vi "main 10th.vi"() -> ()   [LabVIEW 2015]
uses:
  Abort.vi
panel:
  out "OD Num 2":i32
  in  "Direct Summing Cluster":T1={"Direct Summing Path Na"="Nasum9", "Direct Summing Path Rb"="Rbsum9", "Enable Summing"=[FALSE, FALSE]}
  out "number of function calls":i32=187
  out "External Trigger":bool
  out "x-y":u32
  in  "Live Image Display 2":refnum<k7>(container)
  in  "Live Image Display":refnum<k7>(container)
  in  "Initial guess values 2":dbl[](array[numeric])
  in  "Fitting Results Save Path 2":string[](array[string])
  out "Current File Num":u16
  out "Two Cameras ?":bool
  out "3":u32=2150809629
  out "2":u32=2150809629
  out "5":u32=2150809629
  out "4":u32=2150809629
  out "From OD fit?":bool
  in  "Fitting Results Save Path":string[](array[string])
  in  "Initial guess values":dbl[](array[numeric])
  out "Latest image data":dbl[][](array[numeric])
  in  "Fitting Type":u16(ring)
  in  "Force Guess?":bool
  in  "Tab Control":enum32{"Page 1", "Page 2"}(tab)
  in  "Na Fitting ROI":T2
  in  "Rb Fitting ROI":T2
  in  "Get Image":bool
  in  "Open Na/Rb":u16(ring)=1 items=["Na", "Rb"]
  in  "Na/Rb (0/1)":u8(ring) items=["Na", "Rb"]
  in  "Abort":bool
  in  "FFT Auto?":bool[](array[boolean])=[FALSE, FALSE] caption="Auto?"
  in  "Ring":u16(ring)=3 items=["Atom", "Light", "Dark", "OD"]
  in  "Select Cam Fit":bool[](array[boolean])=[FALSE, FALSE]
  in  "Binning Average?":bool caption="Average?"
  in  "FFT Process":bool caption="Process"
  in  "Threshold":dbl
  out "Label":string[](array[string])=["Peak", "Xc", "Yc", "SigX", "SigY", "Offset"]
  in  "Pics to show in IJ":bool[][](array[boolean])=[[FALSE, FALSE], [FALSE, FALSE], [FALSE, FALSE], [TRUE, TRUE]]
  out "Trigger":bool
  in  "Save Fit":bool
  out "best fit parameters 2":dbl[][](array[numeric])
  in  "Binning Enabled":bool=TRUE
  in  "Binning":u8[](array[numeric])=[2, 2]
  out "ROI Width":u16[](array[numeric])
  out "ROI Height":u16[](array[numeric])
  out "best fit parameters":dbl[][](array[numeric])
  in  "Reset Cam Buffer":bool
  out "OD image":dbl[][](graph)
  out "Vertical Fitting":cluster{i32[], dbl[]}[](graph)
  in  "OD fit":bool caption="Open"
  in  "OD Num":i32
  out "Fitting...":bool
  in  "Exit":bool
  out "Horizontal Fitting":cluster{i32[], dbl[]}[](graph)=[{[0, 1, 2, 3, 4, 5, 6, 7, 8, 9, 10, 11, 12, 13, 14, 15, 16, 17, 18, 19, 20, 21, 22, 23, 24, 25, 26, 27, 28, 29, 30, 31, 32, 33, 34, 35, 36, 37, 38, 39, 40, 41, 42, 43, 44, 45, 46, 47, 48, 49, 50, 51, 52, 53, 54, 55, 56, 57, 58, 59, 60, 61, 62, 63, 64, 65, 66, 67, 68, 69, 70, 71, 72, 73, 74, 75, 76, 77, 78, 79, 80, 81, 82, 83, 84, 85, 86, 87, 88, 89, 90, 91, 92, 93, 94, 95, 96, 97, 98, 99, 100, 101, 102, 103, 104, 105, 106, 107, 108, 109, 110, 111, 112, 113, 114, 115, 116, 117, 118, 119, 120, 121, 122, 123, 124, 125, 126, 127, 128, 129, 130, 131, 132, 133, 134, 135, 136, 137, 138, 139, 140, 141, 142, 143, 144, 145, 146, 147, 148, 149, 150, 151, 152, 153, 154, 155, 156, 157, 158, 159, 160, 161, 162, 163, 164, 165, 166, 167, 168, 169, 170, 171, 172, 173, 174, 175, 176, 177, 178, 179, 180, 181, 182, 183, 184, 185, 186, 187, 188, 189, 190, 191, 192, 193, 194, 195, 196, 197, 198, 199], [271.0, 251.0, 239.0, 241.0, 236.0, 262.0, 271.0, 264.0, 266.0, 276.0, 292.0, 228.0, 254.0, 281.0, 219.0, 235.0, 280.0, 281.0, 291.0, 273.0, 299.0, 232.0, 255.0, 240.0, 222.0, 240.0, 240.0, 279.0, 296.0, 297.0, 339.0, 331.0, 313.0, 319.0, 271.0, 292.0, 320.0, 329.0, 342.0, 366.0, 378.0, 346.0, 370.0, 337.0, 334.0, 380.0, 391.0, 444.0, 455.0, 496.0, 509.0, 523.0, 587.0, 603.0, 674.0, 719.0, 851.0, 957.0, 1087.0, 1198.0, 1344.0, 1496.0, 1728.0, 1883.0, 2195.0, 2355.0, 2618.0, 2793.0, 3092.0, 3461.0, 3553.0, 3556.0, 3917.0, 4123.0, 4392.0, 4166.0, 4433.0, 4167.0, 4185.0, 3907.0, 3845.0, 3513.0, 3349.0, 3193.0, 2986.0, 2742.0, 2439.0, 2364.0, 2228.0, 2124.0, 2115.0, 1979.0, 1826.0, 1691.0, 1515.0, 1349.0, 1218.0, 1097.0, 1000.0, 932.0, 787.0, 729.0, 689.0, 578.0, 552.0, 477.0, 513.0, 476.0, 454.0, 434.0, 426.0, 416.0, 377.0, 352.0, 301.0, 326.0, 343.0, 299.0, 311.0, 312.0, 333.0, 330.0, 327.0, 244.0, 229.0, 253.0, 246.0, 250.0, 212.0, 284.0, 270.0, 266.0, 272.0, 267.0, 277.0, 267.0, 251.0, 272.0, 266.0, 265.0, 217.0, 267.0, 275.0, 261.0, 260.0, 253.0, 240.0, 211.0, 261.0, 288.0, 216.0, 259.0, 250.0, 263.0, 252.0, 231.0, 253.0, 269.0, 246.0, 219.0, 238.0, 279.0, 310.0, 259.0, 238.0, 270.0, 237.0, 224.0, 265.0, 263.0, 237.0, 243.0, 236.0, 287.0, 272.0, 238.0, 270.0, 249.0, 228.0, 276.0, 254.0, 251.0, 258.0, 284.0, 232.0, 275.0, 264.0, 230.0, 206.0, 247.0, 249.0, 299.0, 232.0, 226.0, 274.0, 258.0, 228.0, 237.0, 226.0, 272.0]}, {[0, 1, 2, 3, 4, 5, 6, 7, 8, 9, 10, 11, 12, 13, 14, 15, 16, 17, 18, 19, 20, 21, 22, 23, 24, 25, 26, 27, 28, 29, 30, 31, 32, 33, 34, 35, 36, 37, 38, 39, 40, 41, 42, 43, 44, 45, 46, 47, 48, 49, 50, 51, 52, 53, 54, 55, 56, 57, 58, 59, 60, 61, 62, 63, 64, 65, 66, 67, 68, 69, 70, 71, 72, 73, 74, 75, 76, 77, 78, 79, 80, 81, 82, 83, 84, 85, 86, 87, 88, 89, 90, 91, 92, 93, 94, 95, 96, 97, 98, 99, 100, 101, 102, 103, 104, 105, 106, 107, 108, 109, 110, 111, 112, 113, 114, 115, 116, 117, 118, 119, 120, 121, 122, 123, 124, 125, 126, 127, 128, 129, 130, 131, 132, 133, 134, 135, 136, 137, 138, 139, 140, 141, 142, 143, 144, 145, 146, 147, 148, 149, 150, 151, 152, 153, 154, 155, 156, 157, 158, 159, 160, 161, 162, 163, 164, 165, 166, 167, 168, 169, 170, 171, 172, 173, 174, 175, 176, 177, 178, 179, 180, 181, 182, 183, 184, 185, 186, 187, 188, 189, 190, 191, 192, 193, 194, 195, 196, 197, 198, 199], [258.6806156316728, 258.6716342989377, 258.6626530747521, 258.6536720452062, 258.644691361713, 258.6357112882564, 258.6267322810702, 258.61775512175285, 258.608781137568, 258.59981256259033, 258.5908531241233, 258.58190898580693, 258.57299024978414, 258.56411332615136, 258.5553046339484, 258.54660632509234, 258.53808504915014, 258.5298452400012, 258.5220490536178, 258.5149459806351, 258.5089163736844, 258.50453475825293, 258.5026609419198, 258.50456971619576, 258.5121334787082, 258.52807650614886, 258.556324973247, 258.6024831881351, 258.67447387274734, 258.78338851820223, 258.94460259167346, 259.17921915836735, 259.51591254856515, 259.993249982826, 260.6625721744371, 261.5915121253092, 262.86822258072306, 264.606364643175, 266.95088051361154, 270.08453000321674, 274.2351115263941, 279.6832126987842, 286.77024355158215, 295.9063984703781, 307.5780750260748, 322.3541549900494, 340.8904336545859, 363.9313792544649, 392.3083281288412, 426.93318811176084, 468.7867478105236, 518.9007873197883, 578.3333683044344, 648.1369555436747, 729.3193888427367, 822.7981764748481, 929.3491024699478, 1049.550703700878, 1183.72674293613, 1331.889336934238, 1493.6858449827125, 1668.352932109982, 1854.6813445196683, 2050.994832619432, 2255.1463024696804, 2464.533660376819, 2676.1369496341113, 2886.5772978639948, 3092.1969553318745, 3289.15838608278, 3473.5590667034103, 3641.557451626854, 3789.5045781946988, 3914.0750983875137, 4012.3912077845603, 4082.133040191528, 4121.629620994105, 4129.925401766357, 4106.818677312171, 4052.869728621802, 3969.378232753251, 3858.331211349985, 3722.32442841007, 3564.4615781318566, 3388.236726522453, 3197.4062138342942, 2995.8565487684205, 2787.4747242211, 2576.026886168148, 2365.0504495856335, 2157.7636585036757, 1956.9953263662687, 1765.1361682792287, 1584.1118454713421, 1415.3766700512429, 1259.925933154814, 1118.3240687125547, 990.7453722391384, 877.0237608957168, 776.70806955959, 689.1195940765085, 613.4089728479037, 548.609991424882, 493.6884511769152, 447.5848152437265, 409.24989248464567, 377.67331147174724, 351.90494998495853, 331.0698089332847, 314.3770499408072, 301.12405712687945, 290.6964455185657, 282.56493430017093, 276.2799477549777, 271.46471553103595, 267.80753099497196, 265.05370427973, 262.9976251657801, 261.47523759206035, 260.3571273330433, 259.54233995504075, 258.9529785017419, 258.5295789767464, 258.2272251324483, 258.01234029108025, 257.8600805980793, 257.75224890635894, 257.6756492398139, 257.6208065847789, 257.5809840355968, 257.55143783992105, 257.5288597354012, 257.5109645077476, 257.49618853007837, 257.4834719474245, 257.47210306669035, 257.4616084138856, 257.45167589964194, 257.44210169672607, 257.4327538988841, 257.42354791849357, 257.4144300024347, 257.4053662996607, 257.3963356836851, 257.3873250872788, 257.37832650004066, 257.3693350550716, 257.3603478215476, 257.3513630501138, 257.34237970580045, 257.3333971816626, 257.32441512488083, 257.3154333321509, 257.306451687344, 257.29747012470295, 257.2884886073164, 257.2795071146445, 257.2705256353558, 257.26154416325335, 257.25256269497714, 257.24358122872104, 257.23459976352257, 257.2256182988732, 257.21663683450635, 257.2076553702838, 257.19867390613433, 257.1896924420215, 257.18071097792694, 257.17172951384134, 257.16274804976024, 257.15376658568124, 257.1447851216032, 257.13580365752574, 257.12682219344845, 257.11784072937127, 257.10885926529426, 257.09987780121713, 257.09089633714007, 257.081914873063, 257.07293340898593, 257.06395194490887, 257.0549704808318, 257.0459890167548, 257.0370075526777, 257.02802608860065, 257.0190446245236, 257.0100631604465, 257.00108169636945, 256.9921002322924, 256.9831187682154, 256.9741373041383, 256.96515584006124, 256.9561743759842, 256.9471929119071, 256.93821144783004, 256.92922998375303, 256.92024851967597, 256.9112670555989, 256.90228559152183, 256.89330412744476]}]
  in  "Fit":bool
  in  "Open File":bool
  in  "Auto Fit":bool
  in  "Stop":bool
  in  "Aquire":bool
  in  "Fitting Config":bool
  in  "Camera Config":bool
  in  "Initialize":bool
  # "Cam1"
  # "Cam2"
  # "Atom"
  # "Light"
  # "Dark"
  # "OD"
  # "FFT and Low Pass"
  # "Na"
  # "Rb"
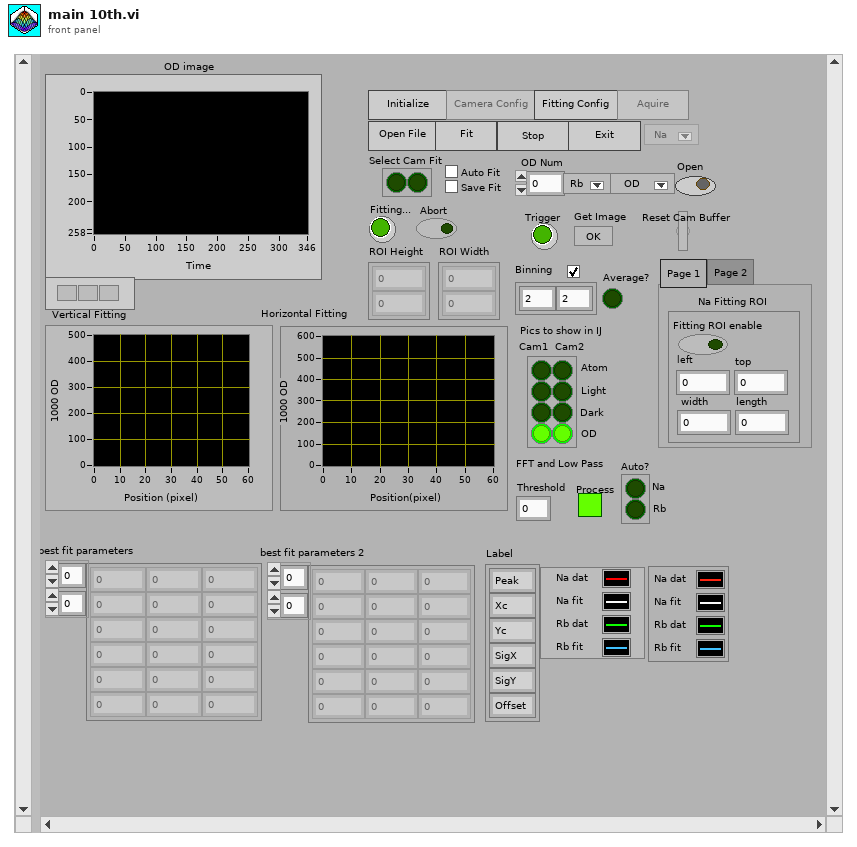
[diagram p1: front panel]
types:
  T1 = cluster{"Direct Summing Path Na":string, "Direct Summing Path Rb":string, "Enable Summing":bool[]}
  T2 = cluster{"Fitting ROI enable":bool, "top":i32, "length":i32, "left":i32, " width":i32}
  T3 = enum8{"Enabled", "Disabled", "Disabled and Grayed Out"}
  T4 = enum16{"Left Button", "Center Button", "Right Button", "Window Close"}
  T5 = typedef "Image Type" = u32
  T6 = typedef "IMAQ Image.ctl" = refnum<image>
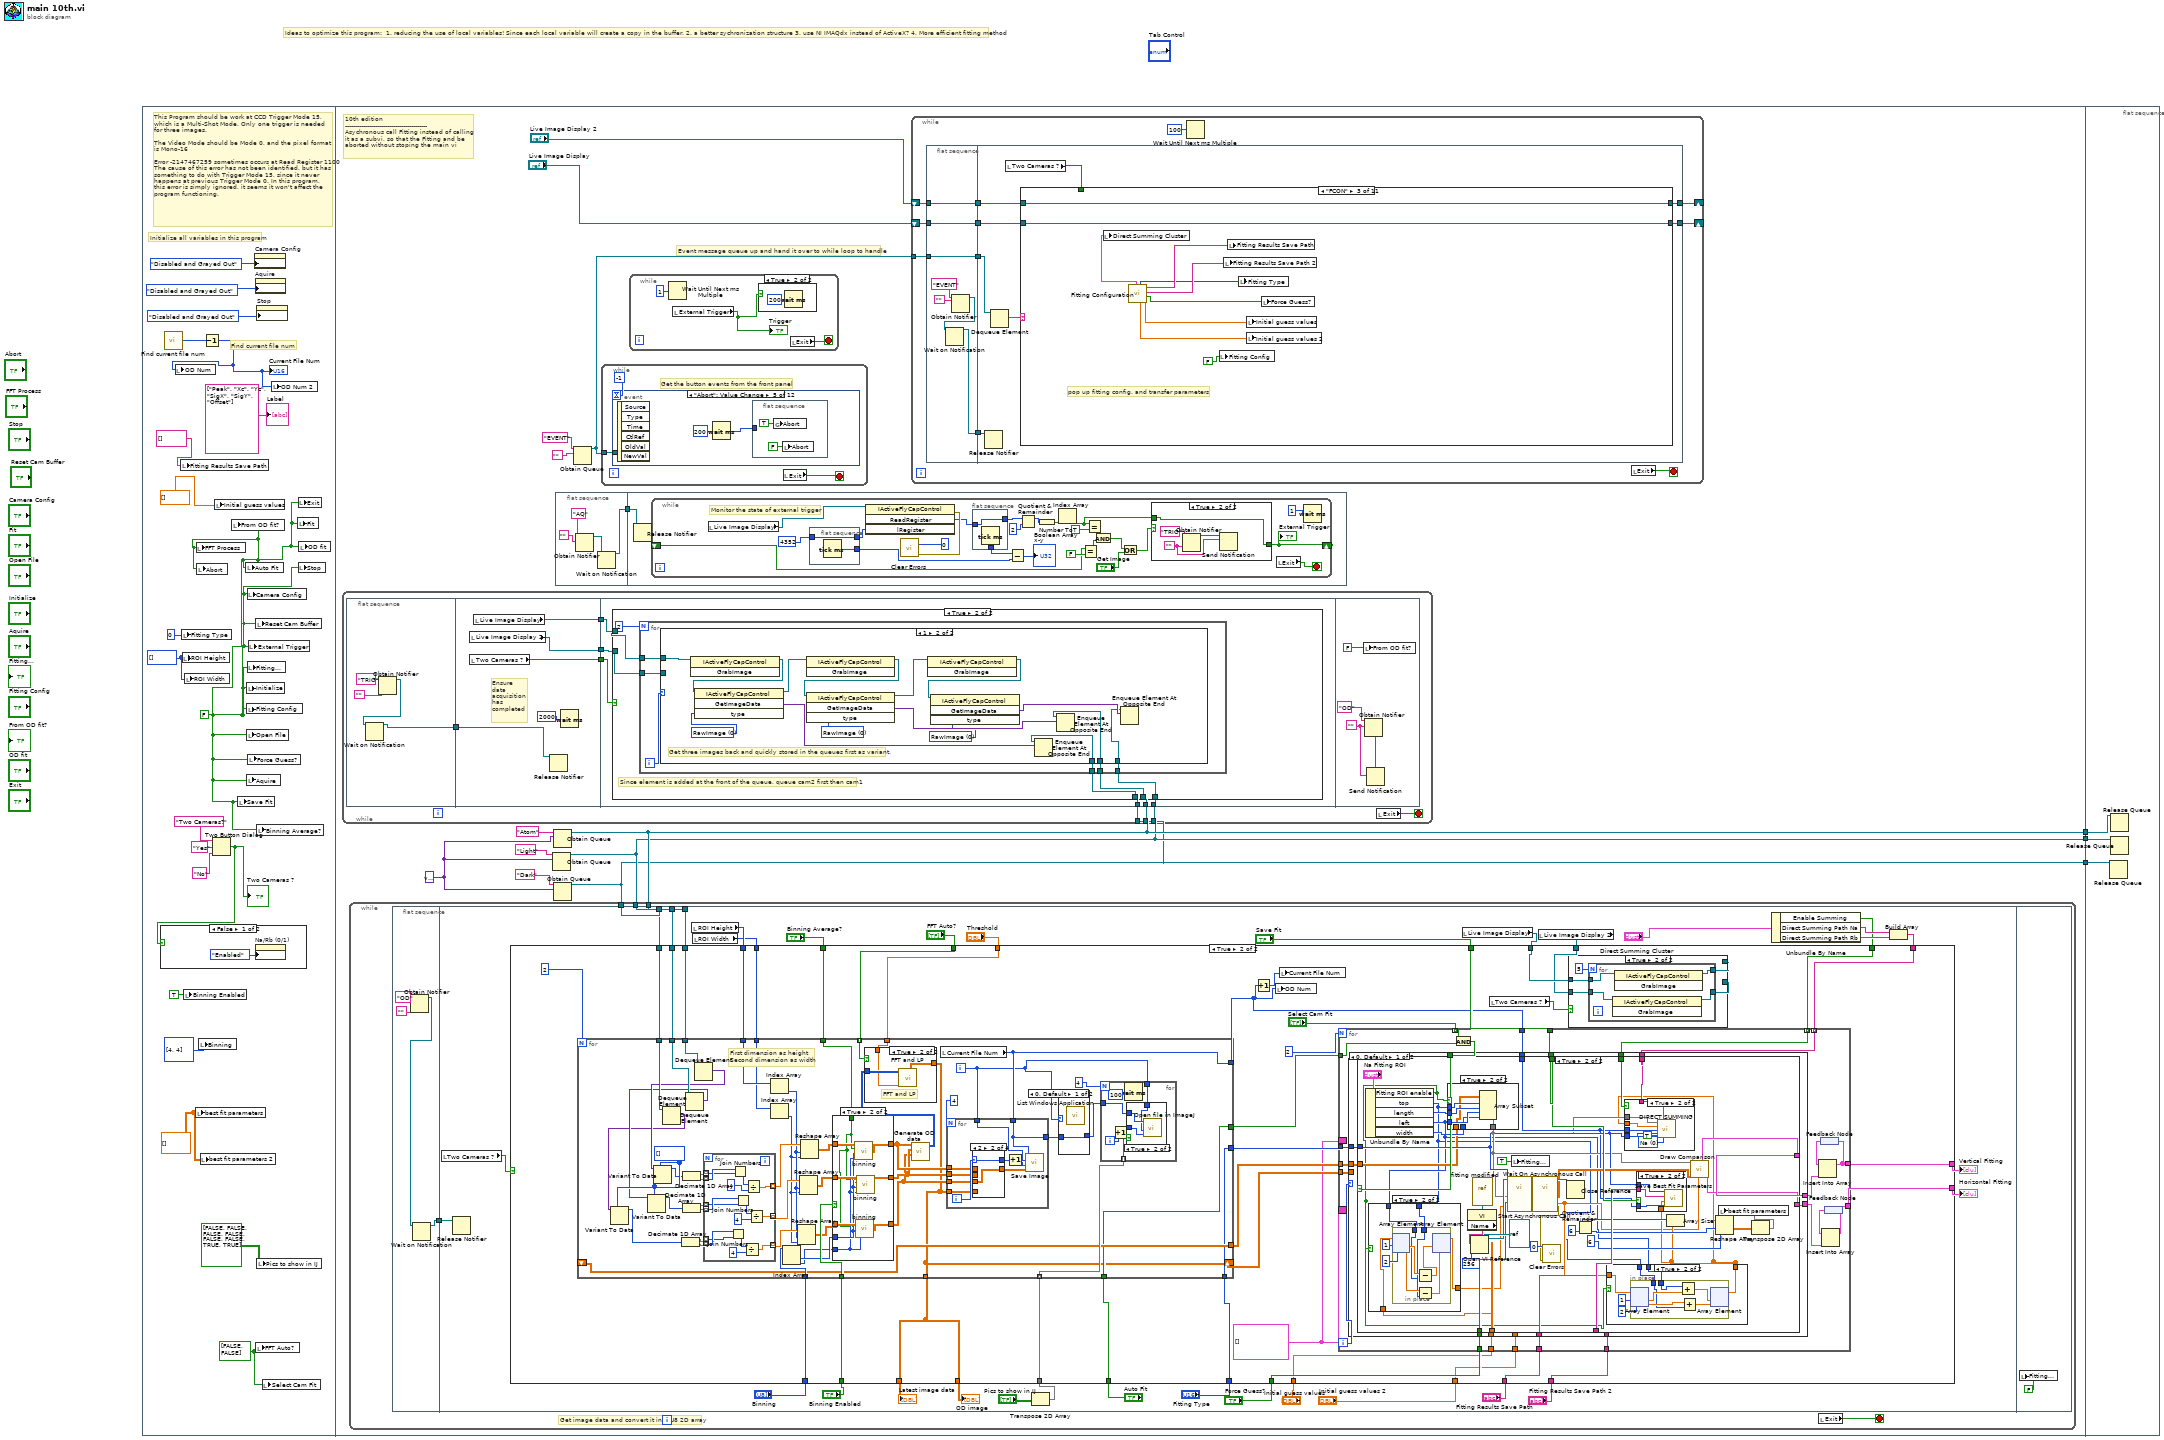
[diagram p0: block diagram]
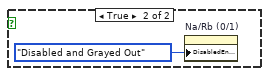
[diagram p2: hidden frame]
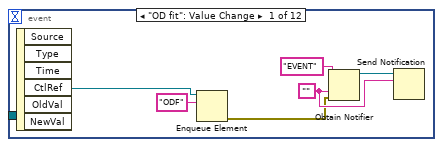
[diagram p4: hidden frame]
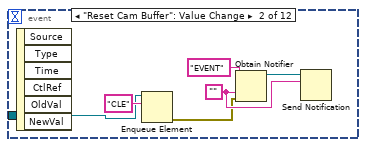
[diagram p5: hidden frame]
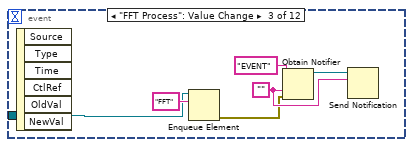
[diagram p6: hidden frame]
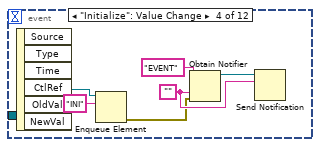
[diagram p7: hidden frame]
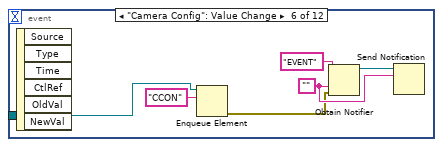
[diagram p8: hidden frame]
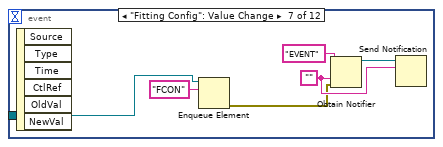
[diagram p9: hidden frame]
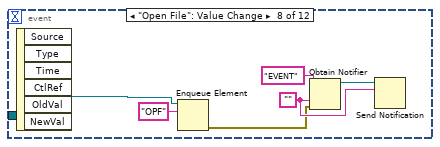
[diagram p10: hidden frame]
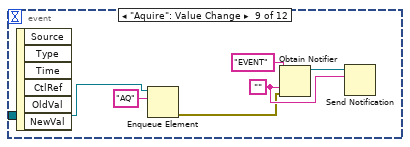
[diagram p11: hidden frame]
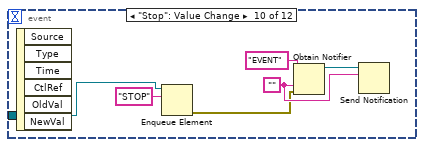
[diagram p12: hidden frame]
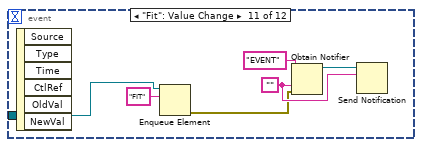
[diagram p13: hidden frame]
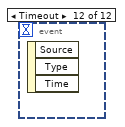
[diagram p14: hidden frame]
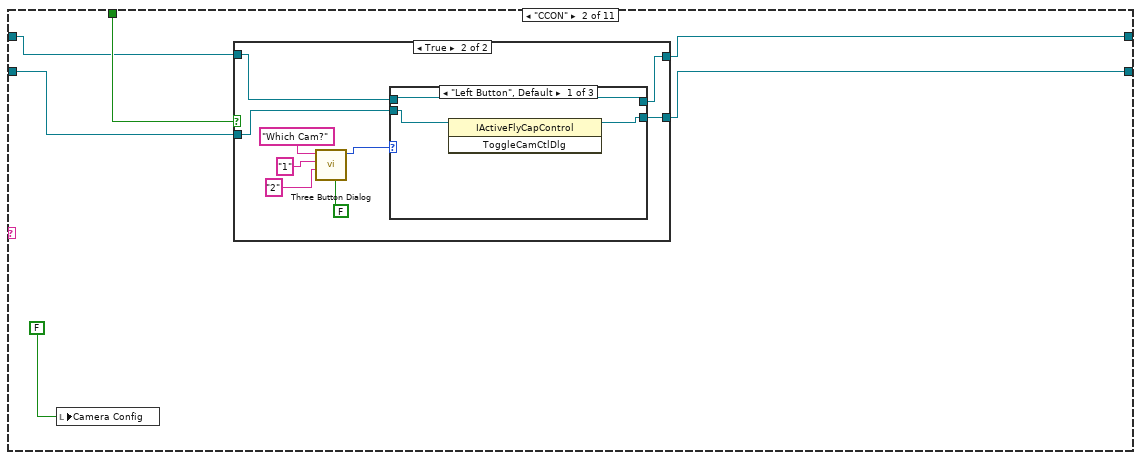
[diagram p16: hidden frame]
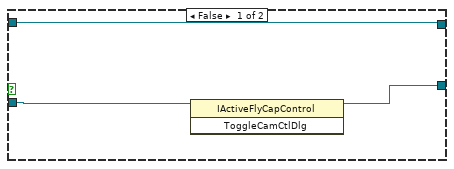
[diagram p17: hidden frame]
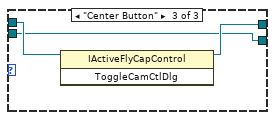
[diagram p19: hidden frame]
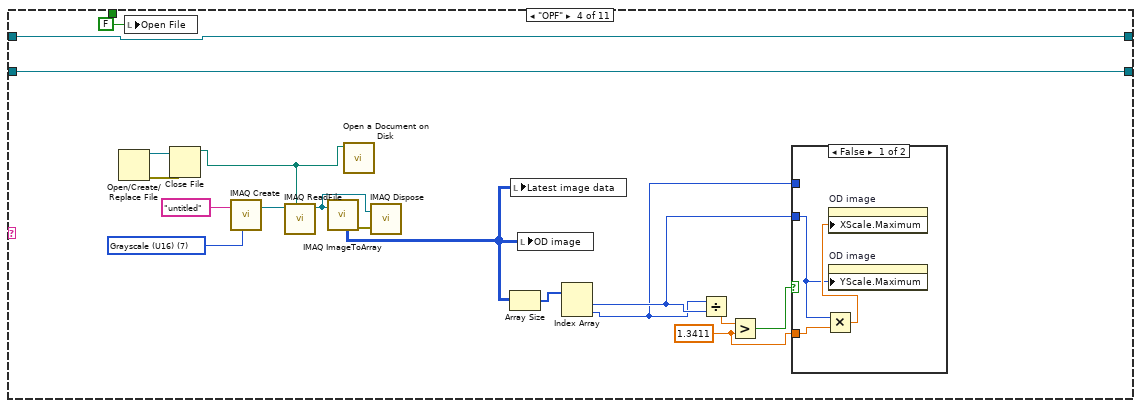
[diagram p20: hidden frame]
diagram:
  # "Ideas to optimize this program:  1. reducing the use of local variables! Since each local variable will create a copy in the buffer. 2. a better sychronization structure 3. use NI IMAQdx instead of ActiveX? 4. More efficient fitting method"
  n1 = flat-sequence {
    tunnel: [w34] -> w3
    tunnel: [w33] -> w2
    tunnel: [w32] -> w1
    tunnel: w3 -> [w1227]
    tunnel: w2 -> [w1226]
    tunnel: w1 -> [w1225]
    frame #0 {
      w5 = bool[] [FALSE, FALSE] ("FFT Auto?")
      w10 = dbl[][] [] ("best fit parameters")
      w14 = u16[] [] ("ROI Height")
      w8 = FALSE ("Aquire")
      # "This Program should be work at CCD Trigger Mode 15,\nwhich is a Multi-Shot Mode. Only one trigger is needed\nfor three images. \n\nThe Video Mode should be Mode 0, and the pixel format\nis Mono-16\n\nError -2147467259 sometimes occurs at Read Register 1100\nThe cause of this error has not been identified, but it has\nsomething to do with Trigger Mode 15, since it never \nhappens at previous Trigger Mode 0. In this program,\nthis error is simply ignored, it seems it won't affect the \nprogram functioning."
      # "Find current file num"
      # "Initialize all variables in this program"
      n2 = call "Find current file num.vi"() -> ("Current File Num"=w9:u16)  [unwired: 2 in]
      n3 = local write "Fitting Results Save Path"(string[] [] ("Fitting Results Save Path")) -> ()
      n4 = local write "Fitting Type"(0 ("OD num")) -> ()
      n5 = local write "ROI Height"(w14) -> ()
      n6 = local write "Binning Enabled"(TRUE ("Binning Enabled")) -> ()
      n7 = local write "ROI Width"(w14) -> ()
      n8 = local write "best fit parameters"(w10) -> ()
      n9 = local write "FFT Process"(w8) -> ()
      n10 = local write "Abort"(w8) -> ()
      n11 = local write "Binning"(u8[] [4, 4] ("Binning")) -> ()
      n12 = local write "best fit parameters 2"(w10) -> ()
      n13 = Decrement(x=w9) -> (x-1=w4:u16)
      "Current File Num" <- w4
      n14 = local write "OD Num"(w4) -> ()
      n15 = Two Button Dialog(message="Two Cameras?" ("消息"), 1:"No" ("F按钮名称（“取消”）"), 2:"Yes" ("T按钮名称（“确定”）")) -> (T button?=w7:bool)
      "Two Cameras ?" <- w7
      n16 = case shown="False" w7 {
        frame False {
          n17 = property on="Na/Rb (0/1)" class="Ring (strict)"("DisabledEnum"=T3."Enabled" ("Disabled")) -> ()  [unwired: 2 in, 2 out]
        }
        frame True {
          n18 = property on="Na/Rb (0/1)" class="Ring (strict)"("DisabledEnum"=T3."Disabled and Grayed Out" ("Disabled")) -> ()  [unwired: 2 in, 2 out]
        }
      }
      n19 = local write "Initial guess values"(dbl[] [] ("Best fit parameters")) -> ()
      n20 = local write "From OD fit?"(w8) -> ()
      n21 = local write "Save Fit"(w8) -> ()
      n22 = local write "Auto Fit"(w8) -> ()
      n23 = local write "Initialize"(w8) -> ()
      n24 = local write "Fitting Config"(w8) -> ()
      n25 = local write "Open File"(w8) -> ()
      n26 = local write "Aquire"(w8) -> ()
      n27 = local write "Camera Config"(w8) -> ()
      n28 = local write "Fitting..."(w8) -> ()
      n29 = local write "Force Guess?"(w8) -> ()
      n30 = local write "External Trigger"(w8) -> ()
      n31 = property on="Camera Config" class="Bool (strict)"("DisabledEnum"=T3."Disabled and Grayed Out" ("禁用")) -> ()  [unwired: 2 in, 2 out]
      n32 = property on="Aquire" class="Bool (strict)"("DisabledEnum"=T3."Disabled and Grayed Out" ("禁用")) -> ()  [unwired: 2 in, 2 out]
      n33 = local write "Reset Cam Buffer"(w8) -> ()
      n34 = local write "FFT Auto?"(w5) -> ()
      n35 = local write "Binning Average?"(w8) -> ()
      n36 = property on="Stop" class="Bool (strict)"("DisabledEnum"=T3."Disabled and Grayed Out" ("禁用")) -> ()  [unwired: 2 in, 2 out]
      n37 = local write "Pics to show in IJ"(bool[][] [[FALSE, FALSE], [FALSE, FALSE], [FALSE, FALSE], [TRUE, TRUE]] ("Pics to show in IJ")) -> ()
      n38 = local write "Select Cam Fit"(w5) -> ()
      n39 = local write "OD Num 2"(w4) -> ()
      n40 = local write "Fit"(w8) -> ()
      n41 = local write "Exit"(w8) -> ()
      n42 = local write "Stop"(w8) -> ()
      n43 = local write "OD fit"(w8) -> ()
      "Label" <- string[] ["Peak", "Xc", "Yc", "SigX", "SigY", "Offset"] ("Label")
    }
    frame #1 {
      w28 = variant
      # "10th edition\n-----------------------------------------\nAsychronous call Fitting instead of calling\nit as a subvi, so that the Fitting and be \naborted without stoping the main vi"
      # "Event message queue up and hand it over to while loop to handle"
      n44 = Obtain Queue(name (unnamed)="Light" ("名称（未命名）"), element data type=w28) -> (queue out=w33:refnum<queue>)  [unwired: 3 in, 2 out]
      n45 = Obtain Queue(name (unnamed)="Atom" ("名称（未命名）"), element data type=w28) -> (queue out=w34:refnum<queue>)  [unwired: 3 in, 2 out]
      n46 = Obtain Queue(name (unnamed)="Dark" ("名称（未命名）"), element data type=w28) -> (queue out=w32:refnum<queue>)  [unwired: 3 in, 2 out]
      n47 = while {
        tunnel: w34 -> [w1135]
        tunnel: w33 -> [w1134]
        tunnel: w32 -> [w1133]
        stop <- w1129 stop-if-true
        n48 = flat-sequence {
          tunnel: [w1137] -> w1136
          tunnel: w1136 -> [w1145]
          tunnel: [w1144] -> w1132
          tunnel: [w1143] -> w1131
          tunnel: [w1142] -> w1130
          tunnel: w1135 -> [w1151]
          tunnel: w1134 -> [w1150]
          tunnel: w1133 -> [w1149]
          tunnel: w1132 -> [w1148]
          tunnel: w1131 -> [w1147]
          tunnel: w1130 -> [w1146]
          frame #0 {
            n49 = Obtain Notifier(name (unnamed)="TRIG" ("名称（未命名）"), notification data type="") -> (notifier out=w1138:refnum<notifier>)  [unwired: 2 in, 2 out]
            n50 = Wait on Notification(notifier=w1138) -> (notifier out=w1137:refnum<notifier>)  [unwired: 3 in, 3 out]
          }
          frame #1 {
            # "Ensure\ndata\nacquisition\nhas \ncompleted"
            n51 = local read "Live Image Display 2"() -> (w1143:refnum<k7>)
            n52 = local read "Two Cameras ?"() -> (w1142:bool)
            n53 = local read "Live Image Display"() -> (w1144:refnum<k7>)
            n54 = Release Notifier(notifier=w1145) -> ()  [unwired: 2 in, 3 out]
            n55 = Wait (ms)(milliseconds to wait=u32 2000) -> ()  [unwired: 1 out]
          }
          frame #2 {
            n56 = case shown="True" w1146 {
              tunnel: w1151 -> [w1169 w1184]
              tunnel: w1150 -> [w1160 w1183]
              tunnel: w1149 -> [w1157 w1182]
              tunnel: w1148 -> [w1153 w1180]
              tunnel: w1147 -> [_ w1179]
              frame False {
                w1155 = 0 items=["RawImage", "ColorProcessedImage"] ("type")
                w1156 = 0 items=["RawImage", "ColorProcessedImage"] ("type")
                w1170 = 0 items=["RawImage", "ColorProcessedImage"] ("type")
                # "Get three images back and quickly stored in the queues first as variant."
                n57 = invoke class="IActiveFlyCapControl" method="GrabImage"(reference=w1153) -> (reference out=w1152:refnum<k7>)  [unwired: 2 in, 2 out]
                n58 = flat-sequence {
                  tunnel: w1152 -> [w1173]
                  tunnel: [w1173] -> w1167
                  frame #0 {
                    n59 = Tick Count (ms)() -> (millisecond timer value=→"2":u32)
                  }
                }
                n60 = invoke class="IActiveFlyCapControl" method="GetImageData"(reference=w1167, "type"=w1170) -> (reference out=w1164:refnum<k7>, "GetImageData"=w1166:variant)  [unwired: 2 in, 2 out]
                n61 = invoke class="IActiveFlyCapControl" method="GrabImage"(reference=w1164) -> (reference out=w1163:refnum<k7>)  [unwired: 2 in, 2 out]
                n62 = flat-sequence {
                  tunnel: [w1171] -> w1165
                  tunnel: w1166 -> [w1171]
                  frame #0 {
                    n63 = Tick Count (ms)() -> (millisecond timer value=→"3":u32)
                  }
                }
                n64 = invoke class="IActiveFlyCapControl" method="GetImageData"(reference=w1163, "type"=w1156) -> (reference out=w1162:refnum<k7>, "GetImageData"=w1161:variant)  [unwired: 2 in, 2 out]
                n65 = flat-sequence {
                  tunnel: w1165 -> [w1178]
                  tunnel: [w1178] -> w1168
                  frame #0 {
                    n66 = Tick Count (ms)() -> (millisecond timer value=→"4":u32)
                  }
                }
                n67 = invoke class="IActiveFlyCapControl" method="GrabImage"(reference=w1162) -> (reference out=w1159:refnum<k7>)  [unwired: 2 in, 2 out]
                n68 = Enqueue Element At Opposite End(queue=w1169, element=w1168) -> ()  [unwired: 2 in, 3 out]
                n69 = Enqueue Element At Opposite End(queue=w1160, element=w1161) -> ()  [unwired: 2 in, 3 out]
                n70 = invoke class="IActiveFlyCapControl" method="GetImageData"(reference=w1159, "type"=w1155) -> ("GetImageData"=w1158:variant)  [unwired: 2 in, 3 out]
                n71 = flat-sequence {
                  tunnel: w1157 -> [w1175]
                  tunnel: [w1175] -> w1154
                  frame #0 {
                    n72 = Tick Count (ms)() -> (millisecond timer value=→"5":u32)
                  }
                }
                n73 = Enqueue Element At Opposite End(queue=w1154, element=w1158) -> ()  [unwired: 2 in, 3 out]
              }
              frame True {
                # "Since element is added at the front of the queue, queue cam2 first then cam1"
                n74 = for {
                  N: 2 -> [_]
                  tunnel: w1184 -> [w1190]
                  tunnel: w1183 -> [w1189]
                  tunnel: w1182 -> [w1188]
                  tunnel: w1180 -> [w1186]
                  tunnel: w1179 -> [w1185]
                  i -> [w1187]
                  n75 = case shown="1" w1187 {
                    tunnel: w1190 -> [w1194 w1210]
                    tunnel: w1189 -> [w1193 w1209]
                    tunnel: w1188 -> [w1192 w1208]
                    tunnel: w1186 -> [_ w1207]
                    tunnel: w1185 -> [w1191 _]
                    frame 0, Default {
                      w1197 = 0 items=["RawImage", "ColorProcessedImage"] ("type")
                      w1198 = 0 items=["RawImage", "ColorProcessedImage"] ("type")
                      w1205 = 0 items=["RawImage", "ColorProcessedImage"] ("type")
                      # "Get three images back and quickly stored in the queues first as variant."
                      n76 = invoke class="IActiveFlyCapControl" method="GrabImage"(reference=w1191) -> (reference out=w1196:refnum<k7>)  [unwired: 2 in, 2 out]
                      n77 = invoke class="IActiveFlyCapControl" method="GetImageData"(reference=w1196, "type"=w1205) -> (reference out=w1204:refnum<k7>, "GetImageData"=w1195:variant)  [unwired: 2 in, 2 out]
                      n78 = invoke class="IActiveFlyCapControl" method="GrabImage"(reference=w1204) -> (reference out=w1203:refnum<k7>)  [unwired: 2 in, 2 out]
                      n79 = invoke class="IActiveFlyCapControl" method="GetImageData"(reference=w1203, "type"=w1198) -> (reference out=w1202:refnum<k7>, "GetImageData"=w1201:variant)  [unwired: 2 in, 2 out]
                      n80 = invoke class="IActiveFlyCapControl" method="GrabImage"(reference=w1202) -> (reference out=w1200:refnum<k7>)  [unwired: 2 in, 2 out]
                      n81 = invoke class="IActiveFlyCapControl" method="GetImageData"(reference=w1200, "type"=w1197) -> ("GetImageData"=w1199:variant)  [unwired: 2 in, 3 out]
                      n82 = Enqueue Element At Opposite End(queue=w1194, element=w1195) -> ()  [unwired: 2 in, 3 out]
                      n83 = Enqueue Element At Opposite End(queue=w1193, element=w1201) -> ()  [unwired: 2 in, 3 out]
                      n84 = Enqueue Element At Opposite End(queue=w1192, element=w1199) -> ()  [unwired: 2 in, 3 out]
                    }
                    frame 1 {
                      w1213 = 0 items=["RawImage", "ColorProcessedImage"] ("type")
                      w1214 = 0 items=["RawImage", "ColorProcessedImage"] ("type")
                      w1220 = 0 items=["RawImage", "ColorProcessedImage"] ("type")
                      # "Get three images back and quickly stored in the queues first as variant."
                      n85 = invoke class="IActiveFlyCapControl" method="GrabImage"(reference=w1207) -> (reference out=w1212:refnum<k7>)  [unwired: 2 in, 2 out]
                      n86 = invoke class="IActiveFlyCapControl" method="GetImageData"(reference=w1212, "type"=w1220) -> (reference out=w1219:refnum<k7>, "GetImageData"=w1211:variant)  [unwired: 2 in, 2 out]
                      n87 = invoke class="IActiveFlyCapControl" method="GrabImage"(reference=w1219) -> (reference out=w1218:refnum<k7>)  [unwired: 2 in, 2 out]
                      n88 = invoke class="IActiveFlyCapControl" method="GetImageData"(reference=w1218, "type"=w1214) -> (reference out=w1217:refnum<k7>, "GetImageData"=w1216:variant)  [unwired: 2 in, 2 out]
                      n89 = invoke class="IActiveFlyCapControl" method="GrabImage"(reference=w1217) -> (reference out=w1206:refnum<k7>)  [unwired: 2 in, 2 out]
                      n90 = invoke class="IActiveFlyCapControl" method="GetImageData"(reference=w1206, "type"=w1213) -> ("GetImageData"=w1215:variant)  [unwired: 2 in, 3 out]
                      n91 = Enqueue Element At Opposite End(queue=w1210, element=w1211) -> ()  [unwired: 2 in, 3 out]
                      n92 = Enqueue Element At Opposite End(queue=w1209, element=w1216) -> ()  [unwired: 2 in, 3 out]
                      n93 = Enqueue Element At Opposite End(queue=w1208, element=w1215) -> ()  [unwired: 2 in, 3 out]
                    }
                  }
                }
              }
            }
          }
          frame #3 {
            w1222 = ""
            n94 = local write "From OD fit?"(FALSE ("From OD fit?")) -> ()
            n95 = Obtain Notifier(name (unnamed)="OD" ("名称（未命名）"), notification data type=w1222) -> (notifier out=w1224:refnum<notifier>)  [unwired: 2 in, 2 out]
            n96 = Send Notification(notification=w1222, notifier=w1224) -> ()  [unwired: 1 in, 2 out]
          }
        }
        n97 = local read "Exit"() -> (w1129:bool)
      }
      n98 = while {
        tunnel: w34 -> [w482]
        tunnel: w33 -> [w481]
        tunnel: w32 -> [w480]
        stop <- w479 stop-if-true
        # "Get image data and convert it into U8 2D array"
        n99 = flat-sequence {
          tunnel: [w484] -> w483
          tunnel: w483 -> [w517]
          tunnel: w482 -> [w520]
          tunnel: w481 -> [w519]
          tunnel: w480 -> [w518]
          frame #0 {
            n100 = Obtain Notifier(name (unnamed)="OD" ("名称（未命名）"), notification data type="") -> (notifier out=w485:refnum<notifier>)  [unwired: 2 in, 2 out]
            n101 = Wait on Notification(notifier=w485) -> (notifier out=w484:refnum<notifier>)  [unwired: 3 in, 3 out]
          }
          frame #1 {
            n102 = local read "Two Cameras ?"() -> (w516:bool)
            n103 = Release Notifier(notifier=w517) -> ()  [unwired: 2 in, 3 out]
            n104 = local read "ROI Height"() -> (w513:u16[])
            n105 = local read "ROI Width"() -> (w512:u16[])
            n106 = Transpose 2D Array(2D array="Pics to show in IJ") -> (transposed array=w499:bool[][])
            n107 = local read "Live Image Display"() -> (w495:refnum<k7>)
            n108 = local read "Live Image Display 2"() -> (w496:refnum<k7>)
            n109 = Unbundle By Name("Direct Summing Cluster") -> ("Enable Summing"=w489:bool[], "Direct Summing Path Na"=w491:string, "Direct Summing Path Rb"=w490:string)
            n110 = Build Array(w491, w490) -> (w488:string[])
            n111 = case shown="True" w516 {
              selector: w516 -> [w532 _]
              tunnel: w520 -> [w584 w744]
              tunnel: w519 -> [w583 w743]
              tunnel: w518 -> [w582 w742]
              tunnel: "Binning" -> [w551 w741]
              tunnel: "Binning Enabled" -> [w550 w740]
              tunnel: w513 -> [w549 w739]
              tunnel: w512 -> [w548 w738]
              tunnel: [w525 w737] -> w511
              tunnel: [w525 w737] -> w510
              tunnel: "Auto Fit" -> [w547 w736]
              tunnel: "Initial guess values" -> [w546 w725]
              tunnel: "Force Guess?" -> [w545 w726]
              tunnel: "Fitting Type" -> [w544 w735]
              tunnel: "Fitting Results Save Path" -> [w543 w722]
              tunnel: [w541 w718] -> w504
              tunnel: [w540 w717] -> w503
              tunnel: "Fitting Results Save Path 2" -> [_ w721]
              tunnel: "Initial guess values 2" -> [_ w720]
              tunnel: "Save Fit" -> [w539 w724]
              tunnel: w499 -> [w538 w733]
              tunnel: "Binning Average?" -> [w536 w732]
              tunnel: w496 -> [w534 w730]
              tunnel: w495 -> [w533 w731]
              tunnel: "Threshold" -> [w529 w714]
              tunnel: "FFT Auto?" -> [w531 w713]
              tunnel: w489 -> [w524 w709]
              tunnel: w488 -> [w522 w708]
              frame False {
                w567 = u8[] []
                # "FFT and LP"
                # "First dimension as height\nSecond dimension as width"
                # "use the current file num flow to control \nthe sequence, save first and then open files in IJ"
                n112 = Dequeue Element(queue=w582) -> (element=w565:variant)  [unwired: 2 in, 3 out]
                n113 = Variant To Data(type=w567, Variant=w565) -> (data=w562:u8[])  [unwired: 1 in, 1 out]
                n114 = Dequeue Element(queue=w583) -> (element=w566:variant)  [unwired: 2 in, 3 out]
                n115 = Variant To Data(type=w567, Variant=w566) -> (data=w563:u8[])  [unwired: 1 in, 1 out]
                n116 = Decimate 1D Array(w562) -> (w573:u8[], w572:u8[])
                n117 = Dequeue Element(queue=w584) -> (element=w568:variant)  [unwired: 2 in, 3 out]
                n118 = Variant To Data(type=w567, Variant=w568) -> (data=w564:u8[])  [unwired: 1 in, 1 out]
                n119 = Decimate 1D Array(w564) -> (w577:u8[], w576:u8[])
                n120 = Decimate 1D Array(w563) -> (w575:u8[], w574:u8[])
                n121 = for {
                  tunnel: [w631] -> w571 mode=indexing
                  tunnel: w577 -> [w621] mode=indexing
                  tunnel: w576 -> [w622] mode=indexing
                  tunnel: w575 -> [w623] mode=indexing
                  tunnel: w574 -> [w624] mode=indexing
                  tunnel: w573 -> [w625] mode=indexing
                  tunnel: w572 -> [w626] mode=indexing
                  tunnel: [w620] -> w570 mode=indexing
                  tunnel: [w619] -> w569 mode=indexing
                  n122 = Join Numbers(hi=w626, lo=w625) -> ((hi.lo)=w628:u16)
                  n123 = Join Numbers(hi=w622, lo=w621) -> ((hi.lo)=w633:u16)
                  n124 = Join Numbers(hi=w624, lo=w623) -> ((hi.lo)=w630:u16)
                  n125 = Divide(x=w628, y=u16 4) -> (x/y=w619:dbl)
                  n126 = Divide(x=w633, y=u16 4) -> (x/y=w631:dbl)
                  n127 = Divide(x=w630, y=u16 4) -> (x/y=w620:dbl)
                }
                n128 = Index Array(array=w548) -> (element=w560:u16)  [unwired: 1 in]
                n129 = Index Array(array=w549) -> (element=w561:u16)  [unwired: 1 in]
                n130 = Reshape Array(w569, w561, w560) -> (w554:dbl[][])
                n131 = Reshape Array(w570, w561, w560) -> (w556:dbl[][])
                n132 = Reshape Array(w571, w561, w560) -> (w558:dbl[][])
                n133 = Index Array(array=w551) -> (element #1=w553:u8, element #2=w552:u8)  [unwired: 2 in]
                n134 = case shown="True" w550 {
                  tunnel: [w609 w617] -> w559
                  tunnel: w558 -> [w609 w618]
                  tunnel: [w608 w615] -> w557
                  tunnel: w556 -> [w608 w616]
                  tunnel: [w607 w614] -> w555
                  tunnel: w554 -> [w607 w613]
                  tunnel: w553 -> [_ w612]
                  tunnel: w552 -> [_ w611]
                  tunnel: w536 -> [_ w610]
                  frame False {
                  }
                  frame True {
                    n135 = call "binning.vi"("y binning"=w611, "x binning"=w612, "Average?"=w610, "data in"=w618) -> ("data out"=w617:dbl[][])
                    n136 = call "binning.vi"("y binning"=w611, "x binning"=w612, "Average?"=w610, "data in"=w613) -> ("data out"=w614:dbl[][])
                    n137 = call "binning.vi"("y binning"=w611, "x binning"=w612, "Average?"=w610, "data in"=w616) -> ("data out"=w615:dbl[][])
                  }
                }
                n138 = Index Array(array=w531) -> (element=w530:bool)  [unwired: 1 in]
                n139 = call "Generate OD data.vi"("dark"=w555, "light"=w557, "atom"=w559) -> ("OD image"=w526:u16[][])  [unwired: 3 in]
                n140 = case shown="True" w530 {
                  tunnel: w526 -> [w586 w589]
                  tunnel: [w586 w588] -> w525
                  tunnel: w529 -> [_ w587]
                  frame False {
                  }
                  frame True {
                    n141 = call "FFT and LP.vi"("Threshold"=w587, "Data In"=w589) -> ("Data Out"=w588:dbl[][])  [unwired: 9 in]
                  }
                }
                n142 = local read "Current File Num"() -> (w535:u16)
                n143 = for {
                  N: 4 -> [_]
                  tunnel: w559 -> [w698]
                  tunnel: w557 -> [w697]
                  tunnel: w555 -> [w696]
                  tunnel: w525 -> [w695]
                  tunnel: w535 -> [w692]
                  tunnel: [w692] -> w578
                  tunnel: ["Na/Rb (0/1)"] -> w527
                  i -> [w699]
                  n144 = case shown="0, Default" w699 {
                    selector: w699 -> [w701 w703 w705 w707]
                    tunnel: w698 -> [w700 _ _ _]
                    tunnel: w697 -> [_ _ _ w706]
                    tunnel: w696 -> [_ w702 _ _]
                    tunnel: w695 -> [_ _ w704 _]
                    tunnel: [w701 w703 w705 w707] -> w694
                    tunnel: [w700 w702 w704 w706] -> w693
                    frame 0, Default {
                    }
                    frame 2 {
                    }
                    frame 3 {
                    }
                    frame 1 {
                    }
                  }
                  n145 = Increment(x=w694) -> (x+1=w690:i32)
                  n146 = call "Save Image.vi"("Data"=w693, "Na/Rb (0/1)"="Na/Rb (0/1)", "Process Index"=w690, "Current File Num"=w692) -> ()  [unwired: 8 in]
                }
                n147 = Index Array(array=w538) -> (element=w537:bool[])  [unwired: 2 in]
                n148 = for {
                  N: 1 -> [_]
                  tunnel: w578 -> [w635]
                  tunnel: [w635] -> w580
                  tunnel: [w634] -> w528
                  tunnel: w527 -> [w634]
                  n149 = call "List Windows Application.vi"() -> ()  [unwired: 1 in]
                }
                n150 = for {
                  N: 4 -> [_]
                  tunnel: w580 -> [w641]
                  tunnel: w537 -> [w638] mode=indexing
                  tunnel: w528 -> [w636]
                  i -> [w640]
                  n151 = Increment(x=w640) -> (x+1=w637:i32)
                  n152 = case shown="True" w638 {
                    tunnel: w641 -> [_ w644]
                    tunnel: w637 -> [_ w643]
                    tunnel: w636 -> [_ w642]
                    frame False {
                    }
                    frame True {
                      n153 = call "Open file in ImageJ.vi"("Process Index"=w643, "Na/Rb (0/1)"=w642, "Current File Num"=w644) -> ()  [unwired: 9 in]
                    }
                  }
                  n154 = Wait (ms)(milliseconds to wait=u32 100) -> ()  [unwired: 1 out]
                }
                n155 = local write "OD Num"(w535) -> ()
                n156 = Increment(x=w535) -> (x+1=w542:u16)
                n157 = local write "Current File Num"(w542) -> ()
                n158 = case shown="True" w532 {
                  tunnel: w533 -> [w594 w602]
                  tunnel: [w590 w600] -> _
                  tunnel: w534 -> [w592 w599]
                  tunnel: [w593 w598] -> _
                  frame False {
                    n159 = for {
                      N: 5 -> [_]
                      tunnel: [w597] -> w590
                      tunnel: w594 -> [w596]
                      tunnel: [w595] -> w593
                      tunnel: w592 -> [w595]
                      n160 = invoke class="IActiveFlyCapControl" method="GrabImage"(reference=w596) -> (reference out=w597:refnum<k7>)  [unwired: 2 in, 2 out]
                    }
                  }
                  frame True {
                    n161 = for {
                      N: 5 -> [_]
                      tunnel: w602 -> [w606]
                      tunnel: [w605] -> w600
                      tunnel: w599 -> [w604]
                      tunnel: [w603] -> w598
                      n162 = invoke class="IActiveFlyCapControl" method="GrabImage"(reference=w606) -> (reference out=w605:refnum<k7>)  [unwired: 2 in, 2 out]
                      n163 = invoke class="IActiveFlyCapControl" method="GrabImage"(reference=w604) -> (reference out=w603:refnum<k7>)  [unwired: 2 in, 2 out]
                    }
                  }
                }
                n164 = Index Array(array=w524) -> (element=w523:bool)  [unwired: 1 in]
                n165 = Index Array(array=w522) -> (element=w521:string)  [unwired: 1 in]
                n166 = case shown="True" w547 {
                  tunnel: w525 -> [w645 w652]
                  tunnel: w535 -> [_ w650]
                  tunnel: [w648 w678] -> w541
                  tunnel: [w647 w677] -> w540
                  tunnel: w546 -> [_ w666]
                  tunnel: w545 -> [_ w665]
                  tunnel: w544 -> [_ w649]
                  tunnel: w543 -> [_ w672]
                  tunnel: w539 -> [_ w671]
                  tunnel: w523 -> [_ w654]
                  tunnel: w521 -> [_ w653]
                  frame False {
                    n167 = call "Draw Comparison.vi"("Best Fit Parameters"=dbl[] [0.0, 0.0, 0.0, 0.0, 0.0], "Best Fit"=w645, "Raw Data"=w645) -> ("Horizontal Comparison"=w647:cluster{i32[], dbl[]}[], "Vertical Comparison"=w648:cluster{i32[], dbl[]}[])  [unwired: 6 in]
                  }
                  frame True {
                    n168 = vi-ref "fitting modified.vi"() -> (w667:refnum<vi>)
                    n169 = property class="VI"(reference=w667) -> ("Name"=w662:string)  [unwired: 1 in, 2 out]
                    n170 = Open VI Reference(type specifier VI Refnum (for type only)=refnum<vi> refnum, vi path=w662, options=256) -> (vi reference=w664:refnum<vi>)  [unwired: 3 in, 1 out]
                    n171 = local write "Fitting..."(TRUE ("Fitting...")) -> ()
                    n172 = call-by-ref "Start Asynchronous Call"(reference=w664, "fitting type"=w649, "2D data"=w652, "force guess?"=w665, "intial guess value"=w666) -> (reference out=w660:refnum<vi>)  [unwired: 9 in, 5 out]
                    n173 = call-by-ref "Wait On Asynchronous Call"(reference=w660) -> (reference out=w658:refnum<vi>, "number of function calls"=→"number of function calls":i32, "best fit"=w655:dbl[][], "best fit parameters"=w651:dbl[], "error out"=w656:errorcluster)  [unwired: 13 in, 1 out]
                    n174 = Close Reference(reference=w658) -> ()  [unwired: 1 in, 1 out]
                    n175 = Array Size(array=w651) -> (size(s)=w675:i32)
                    n176 = Quotient & Remainder(x=w675, y=6) -> (floor(x/y)=w669:i32)  [unwired: 1 out]
                    n177 = call <vilib>:"Clear Errors.vi"("error in (no error)"=w656, "specific error code to clear (0: all)"=0) -> ()  [unwired: 4 in, 2 out]
                    n178 = Reshape Array(w651, w669, 6 ("dimension size")) -> (w676:dbl[][])
                    n179 = Transpose 2D Array(2D array=w676) -> (transposed array=w670:dbl[][])
                    n180 = case shown="True" w671 {
                      tunnel: w650 -> [_ w689]
                      tunnel: w672 -> [_ w688]
                      tunnel: w651 -> [_ w687]
                      tunnel: w649 -> [_ w686]
                      frame False {
                      }
                      frame True {
                        n181 = call "Save Best Fit Parameters.vi"("Current File Num"=w689, "Best Fit Parameters"=w687, "Fitting Results Save Path"=w688, "Fitting Type"=w686) -> ()  [unwired: 8 in]
                      }
                    }
                    n182 = call "Draw Comparison.vi"("Best Fit Parameters"=w651, "Best Fit"=w655, "Raw Data"=w652) -> ("Horizontal Comparison"=w677:cluster{i32[], dbl[]}[], "Vertical Comparison"=w678:cluster{i32[], dbl[]}[])  [unwired: 6 in]
                    n183 = case shown="True" w654 {
                      tunnel: w649 -> [_ w685]
                      tunnel: w650 -> [_ w684]
                      tunnel: w651 -> [_ w683]
                      tunnel: w652 -> [_ w682]
                      tunnel: w653 -> [_ w681]
                      frame False {
                      }
                      frame True {
                        n184 = local read "Na/Rb (0/1)"() -> (w680:u8)
                        n185 = call "DIRECT SUMMING.vi"("Image Data"=w682, "Fitting Results Save Path"=w681, "Best Fit Parameters"=w683, "File Num"=w684, "Fitting Type"=w685, "Two Cameras?"=FALSE, "Na / Rb"=w680) -> ()  [unwired: 8 in, 1 out]
                      }
                    }
                    n186 = local write "best fit parameters"(w670) -> ()
                  }
                }
              }
              frame True {
                w710 = cluster{i32[], dbl[]}[] []
                n187 = for {
                  N: 2 -> [_]
                  tunnel: w744 -> [w1028]
                  tunnel: w743 -> [w1027]
                  tunnel: w742 -> [w1026]
                  tunnel: w741 -> [w1025]
                  tunnel: w740 -> [w1024]
                  tunnel: w739 -> [w1023]
                  tunnel: w738 -> [w1022]
                  tunnel: [w985] -> w737
                  tunnel: w736 -> [w990]
                  tunnel: w735 -> [w989]
                  tunnel: w733 -> [w1021] mode=indexing
                  tunnel: w732 -> [w1020]
                  shift-right: [w985] -> w711
                  shift-left: _ -> [w991]
                  tunnel: [w991] -> w712
                  tunnel: [w990] -> w727
                  tunnel: [w989] -> w723
                  tunnel: [w988] -> w715
                  tunnel: w714 -> [w986]
                  tunnel: w713 -> [w984] mode=indexing
                  i -> [w983]
                  w1007 = u8[] []
                  # "First dimension as height\nSecond dimension as width"
                  n188 = Dequeue Element(queue=w1026) -> (element=w1005:variant)  [unwired: 2 in, 3 out]
                  n189 = Variant To Data(type=w1007, Variant=w1005) -> (data=w1002:u8[])  [unwired: 1 in, 1 out]
                  n190 = Decimate 1D Array(w1002) -> (w1013:u8[], w1012:u8[])
                  n191 = Dequeue Element(queue=w1027) -> (element=w1006:variant)  [unwired: 2 in, 3 out]
                  n192 = Variant To Data(type=w1007, Variant=w1006) -> (data=w1003:u8[])  [unwired: 1 in, 1 out]
                  n193 = Decimate 1D Array(w1003) -> (w1015:u8[], w1014:u8[])
                  n194 = Dequeue Element(queue=w1028) -> (element=w1008:variant)  [unwired: 2 in, 3 out]
                  n195 = Variant To Data(type=w1007, Variant=w1008) -> (data=w1004:u8[])  [unwired: 1 in, 1 out]
                  n196 = Decimate 1D Array(w1004) -> (w1017:u8[], w1016:u8[])
                  n197 = for {
                    tunnel: [w1059] -> w1011 mode=indexing
                    tunnel: w1017 -> [w1049] mode=indexing
                    tunnel: w1016 -> [w1050] mode=indexing
                    tunnel: w1015 -> [w1051] mode=indexing
                    tunnel: w1014 -> [w1052] mode=indexing
                    tunnel: w1013 -> [w1053] mode=indexing
                    tunnel: w1012 -> [w1054] mode=indexing
                    tunnel: [w1048] -> w1010 mode=indexing
                    tunnel: [w1047] -> w1009 mode=indexing
                    n198 = Join Numbers(hi=w1054, lo=w1053) -> ((hi.lo)=w1056:u16)
                    n199 = Join Numbers(hi=w1050, lo=w1049) -> ((hi.lo)=w1061:u16)
                    n200 = Join Numbers(hi=w1052, lo=w1051) -> ((hi.lo)=w1058:u16)
                    n201 = Divide(x=w1056, y=u16 4) -> (x/y=w1047:dbl)
                    n202 = Divide(x=w1061, y=u16 4) -> (x/y=w1059:dbl)
                    n203 = Divide(x=w1058, y=u16 4) -> (x/y=w1048:dbl)
                  }
                  n204 = Index Array(array=w1022) -> (element=w1000:u16)  [unwired: 1 in]
                  n205 = Index Array(array=w1023) -> (element=w1001:u16)  [unwired: 1 in]
                  n206 = Index Array(array=w1025) -> (element #1=w993:u8, element #2=w992:u8)  [unwired: 2 in]
                  n207 = Reshape Array(w1009, w1001, w1000) -> (w994:dbl[][])
                  n208 = Reshape Array(w1010, w1001, w1000) -> (w996:dbl[][])
                  n209 = Reshape Array(w1011, w1001, w1000) -> (w998:dbl[][])
                  n210 = case shown="True" w1024 {
                    tunnel: [w1037 w1045] -> w999
                    tunnel: w998 -> [w1037 w1046]
                    tunnel: [w1036 w1043] -> w997
                    tunnel: w996 -> [w1036 w1044]
                    tunnel: [w1035 w1042] -> w995
                    tunnel: w994 -> [w1035 w1041]
                    tunnel: w993 -> [_ w1040]
                    tunnel: w992 -> [_ w1039]
                    tunnel: w1020 -> [_ w1038]
                    frame False {
                    }
                    frame True {
                      n211 = call "binning.vi"("y binning"=w1039, "x binning"=w1040, "Average?"=w1038, "data in"=w1046) -> ("data out"=w1045:dbl[][])
                      n212 = call "binning.vi"("y binning"=w1039, "x binning"=w1040, "Average?"=w1038, "data in"=w1041) -> ("data out"=w1042:dbl[][])
                      n213 = call "binning.vi"("y binning"=w1039, "x binning"=w1040, "Average?"=w1038, "data in"=w1044) -> ("data out"=w1043:dbl[][])
                    }
                  }
                  n214 = call "Generate OD data.vi"("dark"=w995, "light"=w997, "atom"=w999) -> ("OD image"=w987:u16[][])  [unwired: 3 in]
                  n215 = case shown="True" w984 {
                    tunnel: w987 -> [w1031 w1034]
                    tunnel: [w1031 w1033] -> w985
                    tunnel: w986 -> [_ w1032]
                    frame False {
                    }
                    frame True {
                      # "FFT and LP"
                      n216 = call "FFT and LP.vi"("Threshold"=w1032, "Data In"=w1034) -> ("Data Out"=w1033:dbl[][])  [unwired: 9 in]
                    }
                  }
                  n217 = local read "Current File Num"() -> (w988:u16)
                  n218 = for {
                    N: 4 -> [_]
                    tunnel: w999 -> [w1079]
                    tunnel: w997 -> [w1078]
                    tunnel: w995 -> [w1077]
                    tunnel: w985 -> [w1076]
                    tunnel: w988 -> [w1073]
                    tunnel: [w1073] -> w981
                    tunnel: w983 -> [w1071]
                    i -> [w1080]
                    n219 = case shown="2" w1080 {
                      selector: w1080 -> [w1082 w1084 w1086 w1088]
                      tunnel: w1079 -> [w1081 _ _ _]
                      tunnel: w1078 -> [_ _ _ w1087]
                      tunnel: w1077 -> [_ w1083 _ _]
                      tunnel: w1076 -> [_ _ w1085 _]
                      tunnel: [w1082 w1084 w1086 w1088] -> w1075
                      tunnel: [w1081 w1083 w1085 w1087] -> w1074
                      frame 0, Default {
                      }
                      frame 2 {
                      }
                      frame 3 {
                      }
                      frame 1 {
                      }
                    }
                    n220 = Increment(x=w1075) -> (x+1=w1072:i32)
                    n221 = call "Save Image.vi"("Data"=w1074, "Na/Rb (0/1)"=w1071, "Process Index"=w1072, "Current File Num"=w1073) -> ()  [unwired: 8 in]
                  }
                  n222 = case shown="0, Default" w983 {
                    tunnel: [w1029 w1030] -> w982
                    tunnel: w981 -> [w1029 w1030]
                    frame 0, Default {
                      n223 = call "List Windows Application.vi"() -> ()  [unwired: 1 in]
                    }
                    frame 1 {
                    }
                  }
                  n224 = for {
                    N: 4 -> [_]
                    tunnel: w982 -> [w1067]
                    tunnel: w1021 -> [w1064] mode=indexing
                    tunnel: w983 -> [w1063]
                    i -> [w1066]
                    n225 = Increment(x=w1066) -> (x+1=w1062:i32)
                    n226 = Wait (ms)(milliseconds to wait=u32 100) -> ()  [unwired: 1 out]
                    n227 = case shown="True" w1064 {
                      tunnel: w1067 -> [_ w1070]
                      tunnel: w1062 -> [_ w1069]
                      tunnel: w1063 -> [_ w1068]
                      frame False {
                      }
                      frame True {
                        n228 = call "Open file in ImageJ.vi"("Process Index"=w1069, "Na/Rb (0/1)"=w1068, "Current File Num"=w1070) -> ()  [unwired: 9 in]
                      }
                    }
                  }
                }
                n229 = Increment(x=w715) -> (x+1=w716:u16)
                n230 = local write "OD Num"(w715) -> ()
                n231 = local write "Current File Num"(w716) -> ()
                n232 = for {
                  N: 2 -> [_]
                  tunnel: "Select Cam Fit" -> [w765] mode=indexing
                  tunnel: w727 -> [w764]
                  tunnel: w712 -> [w762]
                  tunnel: w711 -> [w761]
                  tunnel: w726 -> [w760]
                  tunnel: w725 -> [w759]
                  tunnel: w724 -> [w758]
                  tunnel: w723 -> [w757]
                  tunnel: w722 -> [w756]
                  tunnel: w721 -> [w755]
                  tunnel: w720 -> [w754]
                  tunnel: w715 -> [w753]
                  tunnel: [w750] -> w718
                  tunnel: [w747] -> w717
                  border: w710 -> [_]
                  border: w710 -> [_]
                  tunnel: w709 -> [w746] mode=indexing
                  tunnel: w708 -> [w745] mode=indexing
                  i -> [w766]
                  n233 = And(x=w765, y=w764) -> (x .and. y?=w763:bool)
                  n234 = case shown="0, Default" w766 {
                    tunnel: w763 -> [w771 w877]
                    tunnel: w762 -> [w774 w876]
                    tunnel: w761 -> [_ w875]
                    tunnel: w760 -> [w778 w870]
                    tunnel: w759 -> [w777 _]
                    tunnel: w758 -> [w776 w872]
                    tunnel: w757 -> [w775 w873]
                    tunnel: w756 -> [w773 _]
                    tunnel: w755 -> [_ w874]
                    tunnel: w754 -> [_ w871]
                    tunnel: w753 -> [w772 w869]
                    tunnel: [w769 w868] -> w749
                    tunnel: [w770 w867] -> w751
                    tunnel: w746 -> [w768 w866]
                    tunnel: w745 -> [w767 w865]
                    frame 0, Default {
                      n235 = case shown="True" w771 {
                        tunnel: [w782 w820] -> w770
                        tunnel: [w781 w819] -> w769
                        tunnel: w777 -> [_ w783]
                        tunnel: w778 -> [_ w805]
                        tunnel: w773 -> [_ w818]
                        tunnel: w776 -> [_ w814]
                        tunnel: w775 -> [_ w797]
                        tunnel: w774 -> [w779 w791]
                        tunnel: w772 -> [_ w796]
                        tunnel: w768 -> [_ w798]
                        tunnel: w767 -> [_ w795]
                        frame False {
                          n236 = call "Draw Comparison.vi"("Best Fit Parameters"=dbl[] [0.0, 0.0, 0.0, 0.0, 0.0], "Best Fit"=w779, "Raw Data"=w779) -> ("Horizontal Comparison"=w781:cluster{i32[], dbl[]}[], "Vertical Comparison"=w782:cluster{i32[], dbl[]}[])  [unwired: 6 in]
                        }
                        frame True {
                          n237 = Unbundle By Name("Na Fitting ROI") -> ("Fitting ROI enable"=w784:bool, "top"=w785:i32, "length"=w793:i32, "left"=w786:i32, "width"=w792:i32)
                          n238 = case shown="True" w784 {
                            tunnel: [w834 w838] -> w789
                            tunnel: w786 -> [_ w840]
                            tunnel: w785 -> [_ w839]
                            tunnel: w783 -> [w834 w835]
                            frame False {
                            }
                            frame True {
                              n239 = in-place {
                                in-place-border: w840 -> [w841]
                                in-place-border: w839 -> [w842]
                                n240 = in-place-array #1(w835, 1, 2) -> (w846:dbl, w844:dbl)
                                n241 = Subtract(x=w846, y=w841) -> (x-y=w845:dbl)
                                n242 = Subtract(x=w844, y=w842) -> (x-y=w843:dbl)
                                n243 = in-place-array #1(w845, w843) -> (w838:dbl[])  [unwired: 2 out]
                              }
                            }
                          }
                          n244 = case shown="True" w784 {
                            tunnel: [w847 w853] -> w790
                            tunnel: w785 -> [_ w852]
                            tunnel: w793 -> [_ w851]
                            tunnel: w786 -> [_ w850]
                            tunnel: w792 -> [_ w849]
                            tunnel: w791 -> [w847 w848]
                            frame False {
                            }
                            frame True {
                              n245 = Array Subset(array=w848, index (row)=w852, length (row)=w851, index (col)=w850, length (col)=w849) -> (w853:dbl[][])
                            }
                          }
                          n246 = vi-ref "fitting modified.vi"() -> (w811:refnum<vi>)
                          n247 = property class="VI"(reference=w811) -> ("Name"=w809:string)  [unwired: 1 in, 2 out]
                          n248 = Open VI Reference(type specifier VI Refnum (for type only)=refnum<vi> refnum, vi path=w809, options=256) -> (vi reference=w807:refnum<vi>)  [unwired: 3 in, 1 out]
                          n249 = call-by-ref "Start Asynchronous Call"(reference=w807, "fitting type"=w797, "2D data"=w790, "force guess?"=w805, "intial guess value"=w789) -> (reference out=w806:refnum<vi>)  [unwired: 9 in, 5 out]
                          n250 = local write "Fitting..."(TRUE ("Fitting...")) -> ()
                          n251 = call-by-ref "Wait On Asynchronous Call"(reference=w806) -> (reference out=w804:refnum<vi>, "best fit"=w799:dbl[][], "best fit parameters"=w787:dbl[], "error out"=w802:errorcluster)  [unwired: 13 in, 2 out]
                          n252 = call <vilib>:"Clear Errors.vi"("error in (no error)"=w802, "specific error code to clear (0: all)"=0) -> ()  [unwired: 4 in, 2 out]
                          n253 = Close Reference(reference=w804) -> ()  [unwired: 1 in, 1 out]
                          n254 = case shown="True" w784 {
                            tunnel: w787 -> [w821 w827]
                            tunnel: [w821 w823] -> w788
                            tunnel: w786 -> [_ w826]
                            tunnel: w785 -> [_ w822]
                            frame False {
                            }
                            frame True {
                              n255 = in-place {
                                in-place-border: w822 -> [w829]
                                in-place-border: w826 -> [w828]
                                n256 = in-place-array #2(w827, 1, 2) -> (w832:dbl, w833:dbl)
                                n257 = Add(x=w828, y=w832) -> (x+y=w831:dbl)
                                n258 = Add(x=w833, y=w829) -> (x+y=w830:dbl)
                                n259 = in-place-array #2(w831, w830) -> (w823:dbl[])  [unwired: 2 out]
                              }
                            }
                          }
                          n260 = case shown="True" w798 {
                            tunnel: w797 -> [_ w860]
                            tunnel: w796 -> [_ w859]
                            tunnel: w788 -> [_ w858]
                            tunnel: w790 -> [_ w857]
                            tunnel: w795 -> [_ w856]
                            frame False {
                            }
                            frame True {
                              w855 = u16 0 items=["Na", "Rb"] ("Na / Rb")
                              n261 = call "DIRECT SUMMING.vi"("Image Data"=w857, "Fitting Results Save Path"=w856, "Best Fit Parameters"=w858, "File Num"=w859, "Fitting Type"=w860, "Two Cameras?"=TRUE, "Na / Rb"=w855) -> ()  [unwired: 8 in, 1 out]
                            }
                          }
                          n262 = case shown="True" w814 {
                            tunnel: w796 -> [_ w864]
                            tunnel: w797 -> [_ w863]
                            tunnel: w818 -> [_ w862]
                            tunnel: w788 -> [_ w861]
                            frame False {
                            }
                            frame True {
                              n263 = call "Save Best Fit Parameters.vi"("Current File Num"=w864, "Best Fit Parameters"=w861, "Fitting Results Save Path"=w862, "Fitting Type"=w863) -> ()  [unwired: 8 in]
                            }
                          }
                          n264 = Array Size(array=w788) -> (size(s)=w817:i32)
                          n265 = Quotient & Remainder(x=w817, y=6) -> (floor(x/y)=w812:i32)  [unwired: 1 out]
                          n266 = call "Draw Comparison.vi"("Best Fit Parameters"=w787, "Best Fit"=w799, "Raw Data"=w790) -> ("Horizontal Comparison"=w819:cluster{i32[], dbl[]}[], "Vertical Comparison"=w820:cluster{i32[], dbl[]}[])  [unwired: 6 in]
                          n267 = Reshape Array(w788, w812, 6 ("dimension size")) -> (w801:dbl[][])
                          n268 = Transpose 2D Array(2D array=w801) -> (transposed array=w800:dbl[][])
                          n269 = local write "best fit parameters"(w800) -> ()
                        }
                      }
                    }
                    frame 1 {
                      n270 = case shown="True" w877 {
                        tunnel: w873 -> [_ w894]
                        tunnel: w870 -> [_ w905]
                        tunnel: [w881 w919] -> w867
                        tunnel: [w880 w918] -> w868
                        tunnel: w874 -> [_ w917]
                        tunnel: w871 -> [_ w888]
                        tunnel: w872 -> [_ w912]
                        tunnel: w876 -> [w878 _]
                        tunnel: w875 -> [_ w893]
                        tunnel: w869 -> [_ w895]
                        tunnel: w866 -> [_ w897]
                        tunnel: w865 -> [_ w896]
                        frame False {
                          n271 = call "Draw Comparison.vi"("Best Fit Parameters"=dbl[] [0.0, 0.0, 0.0, 0.0, 0.0], "Best Fit"=w878, "Raw Data"=w878) -> ("Horizontal Comparison"=w880:cluster{i32[], dbl[]}[], "Vertical Comparison"=w881:cluster{i32[], dbl[]}[])  [unwired: 6 in]
                        }
                        frame True {
                          n272 = vi-ref "fitting modified.vi"() -> (w906:refnum<vi>)
                          n273 = property class="VI"(reference=w906) -> ("Name"=w908:string)  [unwired: 1 in, 2 out]
                          n274 = Open VI Reference(type specifier VI Refnum (for type only)=refnum<vi> refnum, vi path=w908, options=256) -> (vi reference=w902:refnum<vi>)  [unwired: 3 in, 1 out]
                          n275 = Unbundle By Name("Rb Fitting ROI") -> ("Fitting ROI enable"=w886:bool, "top"=w883:i32, "length"=w890:i32, "left"=w884:i32, "width"=w889:i32)
                          n276 = case shown="True" w886 {
                            tunnel: w888 -> [w933 w939]
                            tunnel: [w933 w936] -> w887
                            tunnel: w883 -> [_ w938]
                            tunnel: w884 -> [_ w937]
                            frame False {
                            }
                            frame True {
                              n277 = in-place {
                                in-place-border: w938 -> [w940]
                                in-place-border: w937 -> [w941]
                                n278 = in-place-array #3(w939, 1, 2) -> (w945:dbl, w943:dbl)
                                n279 = Subtract(x=w945, y=w941) -> (x-y=w944:dbl)
                                n280 = Subtract(x=w943, y=w940) -> (x-y=w942:dbl)
                                n281 = in-place-array #3(w944, w942) -> (w936:dbl[])  [unwired: 2 out]
                              }
                            }
                          }
                          n282 = case shown="True" w886 {
                            tunnel: w893 -> [w946 w952]
                            tunnel: [w946 w951] -> w892
                            tunnel: w883 -> [_ w950]
                            tunnel: w890 -> [_ w949]
                            tunnel: w884 -> [_ w948]
                            tunnel: w889 -> [_ w947]
                            frame False {
                            }
                            frame True {
                              n283 = Array Subset(array=w952, index (row)=w950, length (row)=w949, index (col)=w948, length (col)=w947) -> (w951:dbl[][])
                            }
                          }
                          n284 = call-by-ref "Start Asynchronous Call"(reference=w902, "fitting type"=w894, "2D data"=w892, "force guess?"=w905, "intial guess value"=w887) -> (reference out=w901:refnum<vi>)  [unwired: 9 in, 5 out]
                          n285 = call-by-ref "Wait On Asynchronous Call"(reference=w901) -> (reference out=w904:refnum<vi>, "best fit"=w898:dbl[][], "best fit parameters"=w882:dbl[], "error out"=w899:errorcluster)  [unwired: 13 in, 2 out]
                          n286 = call <vilib>:"Clear Errors.vi"("error in (no error)"=w899, "specific error code to clear (0: all)"=0) -> ()  [unwired: 4 in, 2 out]
                          n287 = case shown="True" w886 {
                            tunnel: w882 -> [w920 w926]
                            tunnel: [w920 w921] -> w885
                            tunnel: w884 -> [_ w925]
                            tunnel: w883 -> [_ w924]
                            frame False {
                            }
                            frame True {
                              n288 = in-place {
                                in-place-border: w925 -> [w930]
                                in-place-border: w924 -> [w932]
                                n289 = in-place-array #4(w926, 1, 2) -> (w929:dbl, w931:dbl)
                                n290 = Add(x=w930, y=w929) -> (x+y=w928:dbl)
                                n291 = Add(x=w931, y=w932) -> (x+y=w927:dbl)
                                n292 = in-place-array #4(w928, w927) -> (w921:dbl[])  [unwired: 2 out]
                              }
                            }
                          }
                          n293 = Close Reference(reference=w904) -> ()  [unwired: 1 in, 1 out]
                          n294 = case shown="True" w912 {
                            tunnel: w895 -> [_ w963]
                            tunnel: w894 -> [_ w962]
                            tunnel: w917 -> [_ w961]
                            tunnel: w885 -> [_ w960]
                            frame False {
                            }
                            frame True {
                              n295 = call "Save Best Fit Parameters.vi"("Current File Num"=w963, "Best Fit Parameters"=w960, "Fitting Results Save Path"=w961, "Fitting Type"=w962) -> ()  [unwired: 8 in]
                            }
                          }
                          n296 = case shown="True" w897 {
                            tunnel: w894 -> [_ w959]
                            tunnel: w895 -> [_ w958]
                            tunnel: w885 -> [_ w957]
                            tunnel: w892 -> [_ w956]
                            tunnel: w896 -> [_ w955]
                            frame False {
                            }
                            frame True {
                              w954 = u16 1 items=["Na", "Rb"] ("Na / Rb")
                              n297 = call "DIRECT SUMMING.vi"("Image Data"=w956, "Fitting Results Save Path"=w955, "Best Fit Parameters"=w957, "File Num"=w958, "Fitting Type"=w959, "Two Cameras?"=TRUE, "Na / Rb"=w954) -> ()  [unwired: 8 in, 1 out]
                            }
                          }
                          n298 = Array Size(array=w885) -> (size(s)=w915:i32)
                          n299 = local write "Fitting..."(TRUE ("Fitting...")) -> ()
                          n300 = call "Draw Comparison.vi"("Best Fit Parameters"=w882, "Best Fit"=w898, "Raw Data"=w892) -> ("Horizontal Comparison"=w918:cluster{i32[], dbl[]}[], "Vertical Comparison"=w919:cluster{i32[], dbl[]}[])  [unwired: 6 in]
                          n301 = Quotient & Remainder(x=w915, y=6) -> (floor(x/y)=w910:i32)  [unwired: 1 out]
                          n302 = Reshape Array(w885, w910, 6 ("dimension size")) -> (w916:dbl[][])
                          n303 = Transpose 2D Array(2D array=w916) -> (transposed array=→"best fit parameters 2":dbl[][])
                        }
                      }
                    }
                  }
                  n304 = feedback #5() -> (w752:cluster{i32[], dbl[]}[])
                  n305 = Insert Into Array(array=w752, new element=w751) -> (w750:cluster{i32[], dbl[]}[])  [unwired: 1 in]
                  n306 = feedback-in #5(w750) -> ()
                  n307 = feedback #6() -> (w748:cluster{i32[], dbl[]}[])
                  n308 = Insert Into Array(array=w748, new element=w749) -> (w747:cluster{i32[], dbl[]}[])  [unwired: 1 in]
                  n309 = feedback-in #6(w747) -> ()
                }
                n310 = local read "Two Cameras ?"() -> (w719:bool)
                n311 = case shown="True" w719 {
                  tunnel: w730 -> [w968 w976]
                  tunnel: [w964 w974] -> _
                  tunnel: w731 -> [w966 w973]
                  tunnel: [w967 w972] -> _
                  frame False {
                    n312 = for {
                      N: 5 -> [_]
                      tunnel: [w971] -> w964
                      tunnel: w968 -> [w970]
                      tunnel: [w969] -> w967
                      tunnel: w966 -> [w969]
                      n313 = invoke class="IActiveFlyCapControl" method="GrabImage"(reference=w970) -> (reference out=w971:refnum<k7>)  [unwired: 2 in, 2 out]
                    }
                  }
                  frame True {
                    n314 = for {
                      N: 5 -> [_]
                      tunnel: w976 -> [w980]
                      tunnel: [w979] -> w974
                      tunnel: w973 -> [w978]
                      tunnel: [w977] -> w972
                      n315 = invoke class="IActiveFlyCapControl" method="GrabImage"(reference=w980) -> (reference out=w979:refnum<k7>)  [unwired: 2 in, 2 out]
                      n316 = invoke class="IActiveFlyCapControl" method="GrabImage"(reference=w978) -> (reference out=w977:refnum<k7>)  [unwired: 2 in, 2 out]
                    }
                  }
                }
              }
            }
            "Latest image data" <- w511
            "OD image" <- w510
            "Vertical Fitting" <- w504
            "Horizontal Fitting" <- w503
          }
          frame #2 {
            n317 = local write "Fitting..."(FALSE ("Fitting...")) -> ()
          }
        }
        n318 = local read "Exit"() -> (w479:bool)
      }
      n319 = flat-sequence {
        tunnel: [w1090] -> w38
        tunnel: w38 -> [w1094]
        frame #0 {
          n320 = Obtain Notifier(name (unnamed)="AQ" ("名称（未命名）"), notification data type="") -> (notifier out=w1092:refnum<notifier>)  [unwired: 2 in, 2 out]
          n321 = Wait on Notification(notifier=w1092) -> (notifier out=w1090:refnum<notifier>)  [unwired: 3 in, 3 out]
        }
        frame #1 {
          n322 = Release Notifier(notifier=w1094) -> ()  [unwired: 2 in, 3 out]
          n323 = while {
            shift-right: [w1109] -> _
            shift-left: _ -> [w1108]
            stop <- w1098 stop-if-true
            # "Monitor the state of external trigger"
            n324 = local read "Live Image Display"() -> (w1119:refnum<k7>)
            n325 = flat-sequence {
              tunnel: [w1123] -> w1103
              tunnel: u32 4352 ("lRegister") -> [w1123]
              tunnel: [w1122] -> w1100
              frame #0 {
                n326 = Tick Count (ms)() -> (millisecond timer value=w1122:u32)
              }
            }
            n327 = invoke class="IActiveFlyCapControl" method="ReadRegister"(reference=w1119, "lRegister"=w1103) -> (error out=w1107:errorcluster, "ReadRegister"=w1105:u32)  [unwired: 2 in, 2 out]
            n328 = call <vilib>:"Clear Errors.vi"("error in (no error)"=w1107, "specific error code to clear (0: all)"=0) -> ()  [unwired: 4 in, 2 out]
            n329 = flat-sequence {
              tunnel: w1105 -> [w1121]
              tunnel: [w1121] -> w1104
              tunnel: [w1120] -> w1101
              frame #0 {
                n330 = Tick Count (ms)() -> (millisecond timer value=w1120:u32)
              }
            }
            n331 = Subtract(x=w1101, y=w1100) -> (x-y=→"x-y":u32)
            n332 = Quotient & Remainder(x=w1104, y=u32 2) -> (x-y*floor(x/y)=w1117:u32)  [unwired: 1 out]
            n333 = Number To Boolean Array(number=w1117) -> (Boolean array=w1116:bool[])
            n334 = Index Array(array=w1116) -> (element=w1111:bool)  [unwired: 1 in]
            n335 = Equal?(x=w1108, y=FALSE) -> (x = y?=w1113:bool)
            n336 = Equal?(x=w1111, y=TRUE) -> (x = y?=w1112:bool)
            n337 = And(x=w1112, y=w1113) -> (x .and. y?=w1097:bool)
            n338 = Or(x=w1097, y="Get Image") -> (x .or. y?=w1095:bool)
            n339 = case shown="True" w1095 {
              tunnel: w1111 -> [w1124 w1125]
              tunnel: [w1124 w1125] -> w1109
              frame False {
              }
              frame True {
                w1126 = ""
                n340 = Obtain Notifier(name (unnamed)="TRIG" ("名称（未命名）"), notification data type=w1126) -> (notifier out=w1127:refnum<notifier>)  [unwired: 2 in, 2 out]
                n341 = Send Notification(notification=w1126, notifier=w1127) -> ()  [unwired: 1 in, 2 out]
              }
            }
            "External Trigger" <- w1109
            n342 = local read "Exit"() -> (w1098:bool)
            n343 = Wait (ms)(milliseconds to wait=u32 1) -> ()  [unwired: 1 out]
          }
        }
      }
      n344 = Obtain Queue(name (unnamed)="EVENT" ("名称（未命名）"), element data type="") -> (queue out=w29:refnum<queue>)  [unwired: 3 in, 2 out]
      n345 = while {
        tunnel: w29 -> [w44]
        stop <- w43 stop-if-true
        # "Get the button events from the front panel"
        n346 = event shown="[4] \"Abort\": Value Change" {
          selector: _ -> [_ _ _ _ _ _ _ _ _ _ _ _]
          dyn-events: _ -> [_ _ _ _ _ _ _ _ _ _ _ _]
          timeout: -1 -> [_ _ _ _ _ _ _ _ _ _ _ _]
          tunnel: w44 -> [w46 w52 w58 w65 _ w74 w80 w86 w92 w98 w104 _]
          event "OD fit": Value Change {
            w49 = ""
            n347 = event-data() -> ()  [unwired: 1 in, 6 out]
            n348 = Enqueue Element(queue=w46, element="ODF") -> (error out=w47:errorcluster)  [unwired: 2 in, 2 out]
            n349 = Obtain Notifier(name (unnamed)="EVENT" ("名称（未命名）"), notification data type=w49, error in (no error)=w47) -> (notifier out=w50:refnum<notifier>)  [unwired: 1 in, 2 out]
            n350 = Send Notification(notification=w49, notifier=w50) -> ()  [unwired: 1 in, 2 out]
          }
          event "Reset Cam Buffer": Value Change {
            w55 = ""
            n351 = event-data() -> ()  [unwired: 1 in, 6 out]
            n352 = Enqueue Element(queue=w52, element="CLE") -> (error out=w53:errorcluster)  [unwired: 2 in, 2 out]
            n353 = Obtain Notifier(name (unnamed)="EVENT" ("名称（未命名）"), notification data type=w55, error in (no error)=w53) -> (notifier out=w56:refnum<notifier>)  [unwired: 1 in, 2 out]
            n354 = Send Notification(notification=w55, notifier=w56) -> ()  [unwired: 1 in, 2 out]
          }
          event "FFT Process": Value Change {
            w61 = ""
            n355 = event-data() -> ()  [unwired: 1 in, 6 out]
            n356 = Enqueue Element(queue=w58, element="FFT") -> (error out=w59:errorcluster)  [unwired: 2 in, 2 out]
            n357 = Obtain Notifier(name (unnamed)="EVENT" ("名称（未命名）"), notification data type=w61, error in (no error)=w59) -> (notifier out=w62:refnum<notifier>)  [unwired: 1 in, 2 out]
            n358 = Send Notification(notification=w61, notifier=w62) -> ()  [unwired: 1 in, 2 out]
          }
          event "Initialize": Value Change {
            w67 = ""
            n359 = event-data() -> ()  [unwired: 1 in, 6 out]
            n360 = Enqueue Element(queue=w65, element="INI") -> (error out=w64:errorcluster)  [unwired: 2 in, 2 out]
            n361 = Obtain Notifier(name (unnamed)="EVENT" ("名称（未命名）"), notification data type=w67, error in (no error)=w64) -> (notifier out=w68:refnum<notifier>)  [unwired: 1 in, 2 out]
            n362 = Send Notification(notification=w67, notifier=w68) -> ()  [unwired: 1 in, 2 out]
          }
          event "Abort": Value Change {
            n363 = event-data() -> ()  [unwired: 1 in, 6 out]
            n364 = Wait (ms)(milliseconds to wait=u32 200) -> (millisecond timer value=w70:u32)
            n365 = flat-sequence {
              tunnel: w70 -> [_]
              frame #0 {
                n366 = global write "Abort.vi" "Abort"(TRUE ("Abort")) -> ()
                n367 = local write "Abort"(FALSE ("Abort")) -> ()
              }
            }
          }
          event "Camera Config": Value Change {
            w77 = ""
            n368 = event-data() -> ()  [unwired: 1 in, 6 out]
            n369 = Enqueue Element(queue=w74, element="CCON") -> (error out=w75:errorcluster)  [unwired: 2 in, 2 out]
            n370 = Obtain Notifier(name (unnamed)="EVENT" ("名称（未命名）"), notification data type=w77, error in (no error)=w75) -> (notifier out=w78:refnum<notifier>)  [unwired: 1 in, 2 out]
            n371 = Send Notification(notification=w77, notifier=w78) -> ()  [unwired: 1 in, 2 out]
          }
          event "Fitting Config": Value Change {
            w83 = ""
            n372 = event-data() -> ()  [unwired: 1 in, 6 out]
            n373 = Enqueue Element(queue=w80, element="FCON") -> (error out=w81:errorcluster)  [unwired: 2 in, 2 out]
            n374 = Obtain Notifier(name (unnamed)="EVENT" ("名称（未命名）"), notification data type=w83, error in (no error)=w81) -> (notifier out=w84:refnum<notifier>)  [unwired: 1 in, 2 out]
            n375 = Send Notification(notification=w83, notifier=w84) -> ()  [unwired: 1 in, 2 out]
          }
          event "Open File": Value Change {
            w89 = ""
            n376 = event-data() -> ()  [unwired: 1 in, 6 out]
            n377 = Enqueue Element(queue=w86, element="OPF") -> (error out=w87:errorcluster)  [unwired: 2 in, 2 out]
            n378 = Obtain Notifier(name (unnamed)="EVENT" ("名称（未命名）"), notification data type=w89, error in (no error)=w87) -> (notifier out=w90:refnum<notifier>)  [unwired: 1 in, 2 out]
            n379 = Send Notification(notification=w89, notifier=w90) -> ()  [unwired: 1 in, 2 out]
          }
          event "Aquire": Value Change {
            w95 = ""
            n380 = event-data() -> ()  [unwired: 1 in, 6 out]
            n381 = Enqueue Element(queue=w92, element="AQ") -> (error out=w93:errorcluster)  [unwired: 2 in, 2 out]
            n382 = Obtain Notifier(name (unnamed)="EVENT" ("名称（未命名）"), notification data type=w95, error in (no error)=w93) -> (notifier out=w96:refnum<notifier>)  [unwired: 1 in, 2 out]
            n383 = Send Notification(notification=w95, notifier=w96) -> ()  [unwired: 1 in, 2 out]
          }
          event "Stop": Value Change {
            w101 = ""
            n384 = event-data() -> ()  [unwired: 1 in, 6 out]
            n385 = Enqueue Element(queue=w98, element="STOP") -> (error out=w99:errorcluster)  [unwired: 2 in, 2 out]
            n386 = Obtain Notifier(name (unnamed)="EVENT" ("名称（未命名）"), notification data type=w101, error in (no error)=w99) -> (notifier out=w102:refnum<notifier>)  [unwired: 1 in, 2 out]
            n387 = Send Notification(notification=w101, notifier=w102) -> ()  [unwired: 1 in, 2 out]
          }
          event "Fit": Value Change {
            w107 = ""
            n388 = event-data() -> ()  [unwired: 1 in, 6 out]
            n389 = Enqueue Element(queue=w104, element="FIT") -> (error out=w105:errorcluster)  [unwired: 2 in, 2 out]
            n390 = Obtain Notifier(name (unnamed)="EVENT" ("名称（未命名）"), notification data type=w107, error in (no error)=w105) -> (notifier out=w108:refnum<notifier>)  [unwired: 1 in, 2 out]
            n391 = Send Notification(notification=w107, notifier=w108) -> ()  [unwired: 1 in, 2 out]
          }
          event Timeout {
            n392 = event-data() -> ()  [unwired: 1 in, 3 out]
          }
        }
        n393 = local read "Exit"() -> (w43:bool)
      }
      n394 = while {
        stop <- w39 stop-if-true
        n395 = Wait Until Next ms Multiple(millisecond multiple=u32 1) -> ()  [unwired: 1 out]
        n396 = local read "External Trigger"() -> (w40:bool)
        "Trigger" <- w40
        n397 = case shown="True" w40 {
          frame False {
          }
          frame True {
            n398 = Wait (ms)(milliseconds to wait=u32 200) -> ()  [unwired: 1 out]
          }
        }
        n399 = local read "Exit"() -> (w39:bool)
      }
      n400 = while {
        tunnel: w29 -> [w119]
        shift-right: [w115] -> _
        shift-left: "Live Image Display" -> [w116]
        shift-right: [w114] -> _
        shift-left: "Live Image Display 2" -> [w112]
        stop <- w110 stop-if-true
        n401 = flat-sequence {
          tunnel: [w124] -> w120
          tunnel: w119 -> [w123]
          tunnel: [w123] -> w118
          tunnel: [w122] -> w117
          tunnel: w116 -> [w122]
          tunnel: [w121] -> w113
          tunnel: w112 -> [w121]
          tunnel: w120 -> [w135]
          tunnel: w118 -> [w134]
          tunnel: w117 -> [w132]
          tunnel: [w131] -> w115
          tunnel: [w130] -> w114
          tunnel: w113 -> [w129]
          frame #0 {
            n402 = Obtain Notifier(name (unnamed)="EVENT" ("名称（未命名）"), notification data type="") -> (notifier out=w125:refnum<notifier>)  [unwired: 2 in, 2 out]
            n403 = Wait on Notification(notifier=w125) -> (notifier out=w124:refnum<notifier>)  [unwired: 3 in, 3 out]
          }
          frame #1 {
            n404 = Release Notifier(notifier=w135) -> ()  [unwired: 2 in, 3 out]
            n405 = Dequeue Element(queue=w134) -> (element=w133:string)  [unwired: 2 in, 3 out]
            n406 = local read "Two Cameras ?"() -> (w128:bool)
            n407 = case shown="\"FCON\"" w133 {
              tunnel: w132 -> [w137 w142 w172 w182 w200 w224 w288 w298 w372 w429 w461]
              tunnel: [w137 w141 w172 w182 w200 w223 w287 w298 w372 w423 w460] -> w131
              tunnel: [w136 w139 w171 w181 w201 w220 w286 w297 w371 w424 w456] -> w130
              tunnel: w129 -> [w136 w138 w171 w181 w201 w219 w285 w297 w371 w425 w457]
              tunnel: w128 -> [_ w140 _ _ _ w221 w284 _ _ w426 w458]
              frame Default {
              }
              frame "CCON" {
                n408 = local write "Camera Config"(FALSE ("Camera Config")) -> ()
                n409 = case shown="True" w140 {
                  tunnel: w142 -> [w146 w153]
                  tunnel: [w145 w152] -> w141
                  tunnel: [w144 w150] -> w139
                  tunnel: w138 -> [w144 w151]
                  frame False {
                    n410 = invoke class="IActiveFlyCapControl" method="ToggleCamCtlDlg"(reference=w146) -> (reference out=w145:refnum<k7>)  [unwired: 2 in, 2 out]
                  }
                  frame True {
                    n411 = call <vilib>:"Three Button Dialog.vi"("Allow user to close window? (TRUE)"=FALSE, "Center Button Text (\"No\")"="2" ("F按钮名称（“取消”）"), "Left Button Text (\"Yes\")"="1" ("T按钮名称（“确定”）"), "message"="Which Cam?" ("消息")) -> ("Which Button?"=w154:T4)  [unwired: 7 in]
                    n412 = case shown="\"Left Button\", Default" w154 {
                      tunnel: w153 -> [w158 w160 w161]
                      tunnel: [w157 w160 w161] -> w152
                      tunnel: w151 -> [w156 w159 w162]
                      tunnel: [w156 w159 w163] -> w150
                      frame "Left Button", Default {
                        n413 = invoke class="IActiveFlyCapControl" method="ToggleCamCtlDlg"(reference=w158) -> (reference out=w157:refnum<k7>)  [unwired: 2 in, 2 out]
                      }
                      frame "Right Button" {
                      }
                      frame "Center Button" {
                        n414 = invoke class="IActiveFlyCapControl" method="ToggleCamCtlDlg"(reference=w162) -> (reference out=w163:refnum<k7>)  [unwired: 2 in, 2 out]
                      }
                    }
                  }
                }
              }
              frame "FCON" {
                # "pop up fitting config. and transfer parameters"
                n415 = call "Fitting Configuration.vi"() -> ("Na intial guess"=w166:dbl[], "Force Guess?"=w167:bool, "Na Fitting Results Save Path"=w169:string[], "Rb Fitting Results Save Path"=w170:string[], "Rb intial guess"=w165:dbl[], "Fitting Type"=w168:u16, "Direct Summing Cluster"=w164:T1)  [unwired: 5 in]
                n416 = local write "Direct Summing Cluster"(w164) -> ()
                n417 = local write "Fitting Config"(FALSE ("Fitting Config")) -> ()
                n418 = local write "Fitting Results Save Path 2"(w169) -> ()
                n419 = local write "Fitting Results Save Path"(w170) -> ()
                n420 = local write "Fitting Type"(w168) -> ()
                n421 = local write "Initial guess values"(w166) -> ()
                n422 = local write "Initial guess values 2"(w165) -> ()
                n423 = local write "Force Guess?"(w167) -> ()
              }
              frame "OPF" {
                w177 = 1.3411 ("y")
                w184 = T5 7 items=["Grayscale (U8)", "Grayscale (I16)", "Grayscale (SGL)", "Complex (CSG)", "RGB (U32)", "HSL (U32)", "RGB (U64)", "Grayscale (U16)"] ("Image Type")
                n424 = Open/Create/Replace File() -> (refnum out=w190:refnum<file>, error out=w189:errorcluster)  [unwired: 6 in, 1 out]
                n425 = local write "Open File"(FALSE ("Open File")) -> ()
                n426 = Close File(refnum=w190, error in=w189) -> (path=w191:path)  [unwired: 1 out]
                n427 = call "IMAQ Create"("Image Name"="untitled", "Image Type"=w184) -> ("New Image"=w185:T6)  [unwired: 3 in, 1 out]
                n428 = call "IMAQ ReadFile"("File Path"=w191, "Image"=w185) -> ("Image Out"=w186:T6)  [unwired: 5 in, 4 out]
                n429 = call "IMAQ ImageToArray"("Image"=w186) -> ("Image Pixels (U16)"=w174:u16[][], "error out"=w187:errorcluster)  [unwired: 3 in, 3 out]
                n430 = call <vilib>:"Open a Document on Disk.vi"("document path"=w191) -> ()  [unwired: 6 in, 1 out]
                n431 = call "IMAQ Dispose"("Image"=w186, "error in (no error)"=w187) -> ()  [unwired: 4 in, 1 out]
                n432 = Array Size(array=w174) -> (size(s)=w180:i32[])
                n433 = local write "Latest image data"(w174) -> ()
                n434 = local write "OD image"(w174) -> ()
                n435 = Index Array(array=w180) -> (element #1=w176:i32, element #2=w175:i32)  [unwired: 2 in]
                n436 = Divide(x=w175, y=w176) -> (x/y=w179:dbl)
                n437 = Greater?(x=w179, y=w177) -> (0:w178:bool)
                n438 = case shown="False" w178 {
                  tunnel: w176 -> [w192 _]
                  tunnel: w177 -> [w194 w197]
                  tunnel: w175 -> [_ w195]
                  frame False {
                    n439 = Multiply(x=w192, y=w194) -> (x*y=w193:dbl)
                    n440 = property on="OD image" class="IntGraph (strict)"("XScale.Maximum"=w193) -> ()  [unwired: 2 in, 2 out]
                    n441 = property on="OD image" class="IntGraph (strict)"("YScale.Maximum"=w192) -> ()  [unwired: 2 in, 2 out]
                  }
                  frame True {
                    n442 = Divide(x=w195, y=w197) -> (x/y=w196:dbl)
                    n443 = property on="OD image" class="IntGraph (strict)"("XScale.Maximum"=w195) -> ()  [unwired: 2 in, 2 out]
                    n444 = property on="OD image" class="IntGraph (strict)"("YScale.Maximum"=w196) -> ()  [unwired: 2 in, 2 out]
                  }
                }
              }
              frame "FFT" {
                n445 = local read "Latest image data"() -> (w203:dbl[][])
                n446 = local read "Threshold"() -> (w198:dbl)
                n447 = call "FFT and LP.vi"("Threshold"=w198, "Data In"=w203) -> ("Data Out"=w202:dbl[][])  [unwired: 9 in]
                n448 = local write "Latest image data"(w202) -> ()
                n449 = local write "OD image"(w202) -> ()
                n450 = local write "FFT Process"(FALSE ("FFT Process")) -> ()
              }
              frame "AQ" {
                w214 = 1.3411 ("y")
                w229 = ""
                n451 = Obtain Notifier(name (unnamed)="AQ" ("名称（未命名）"), notification data type=w229) -> (notifier out=w228:refnum<notifier>)  [unwired: 2 in, 2 out]
                n452 = case shown="True" w221 {
                  tunnel: w224 -> [w247 w275]
                  tunnel: [w246 w274] -> w223
                  tunnel: [w245 w264] -> w220
                  tunnel: w219 -> [w245 w265]
                  tunnel: [w240 w257] -> w206
                  tunnel: [w241 w258] -> w209
                  frame False {
                    w242 = 0
                    # "Width"
                    # "Height"
                    # "Get Current ROI size"
                    # "Start the camera"
                    n453 = property class="IActiveFlyCapControl"(reference=w247, "Start"=1) -> (reference out=w246:refnum<k7>)  [unwired: 1 in, 1 out]
                    n454 = invoke class="IActiveFlyCapControl" method="ReadRegister"(reference=w247, "lRegister"=u32 8204) -> ("ReadRegister"=w249:u32)  [unwired: 2 in, 3 out]
                    n455 = Number To Hexadecimal String(2:w249) -> (0:w253:string)  [unwired: 1 in]
                    n456 = String Length(string=w253) -> (length=w250:i32)
                    n457 = Subtract(x=w250, y=4) -> (x-y=w252:i32)
                    n458 = String Subset(string=w253, offset (0)=w252) -> (substring=w254:string)  [unwired: 1 in]
                    n459 = String Subset(string=w253, length (rest)=w252) -> (substring=w255:string)  [unwired: 1 in]
                    n460 = Hexadecimal String To Number(string=w254) -> (number=w243:u32)  [unwired: 2 in, 1 out]
                    n461 = Hexadecimal String To Number(string=w255) -> (number=w244:u32)  [unwired: 2 in, 1 out]
                    n462 = Build Array(w243, w242) -> (w241:u32[])
                    n463 = Build Array(w244, w242) -> (w240:u32[])
                  }
                  frame True {
                    w266 = 1 ("Start")
                    # "Width"
                    # "Get Current ROI size"
                    # "Width"
                    # "Height"
                    # "Get Current ROI size"
                    # "Start the camera"
                    n464 = invoke class="IActiveFlyCapControl" method="ReadRegister"(reference=w275, "lRegister"=u32 8204) -> ("ReadRegister"=w277:u32)  [unwired: 2 in, 3 out]
                    n465 = invoke class="IActiveFlyCapControl" method="ReadRegister"(reference=w265, "lRegister"=u32 8204) -> ("ReadRegister"=w269:u32)  [unwired: 2 in, 3 out]
                    n466 = property class="IActiveFlyCapControl"(reference=w265, "Start"=w266) -> (reference out=w264:refnum<k7>)  [unwired: 1 in, 1 out]
                    n467 = property class="IActiveFlyCapControl"(reference=w275, "Start"=w266) -> (reference out=w274:refnum<k7>)  [unwired: 1 in, 1 out]
                    n468 = Number To Hexadecimal String(2:w277) -> (0:w281:string)  [unwired: 1 in]
                    n469 = Number To Hexadecimal String(2:w269) -> (0:w267:string)  [unwired: 1 in]
                    n470 = String Length(string=w281) -> (length=w278:i32)
                    n471 = String Length(string=w267) -> (length=w270:i32)
                    n472 = Subtract(x=w278, y=4) -> (x-y=w280:i32)
                    n473 = Subtract(x=w270, y=4) -> (x-y=w272:i32)
                    n474 = String Subset(string=w281, offset (0)=w280) -> (substring=w282:string)  [unwired: 1 in]
                    n475 = String Subset(string=w281, length (rest)=w280) -> (substring=w283:string)  [unwired: 1 in]
                    n476 = String Subset(string=w267, offset (0)=w272) -> (substring=w263:string)  [unwired: 1 in]
                    n477 = String Subset(string=w267, length (rest)=w272) -> (substring=w273:string)  [unwired: 1 in]
                    n478 = Hexadecimal String To Number(string=w282) -> (number=w262:u32)  [unwired: 2 in, 1 out]
                    n479 = Hexadecimal String To Number(string=w283) -> (number=w260:u32)  [unwired: 2 in, 1 out]
                    n480 = Hexadecimal String To Number(string=w263) -> (number=w261:u32)  [unwired: 2 in, 1 out]
                    n481 = Hexadecimal String To Number(string=w273) -> (number=w259:u32)  [unwired: 2 in, 1 out]
                    n482 = Build Array(w262, w261) -> (w258:u32[])
                    n483 = Build Array(w260, w259) -> (w257:u32[])
                  }
                }
                "ROI Height" <- w209
                "ROI Width" <- w206
                n484 = Send Notification(notification=w229, notifier=w228) -> ()  [unwired: 1 in, 2 out]
                n485 = property on="Stop" class="Bool (strict)"("DisabledEnum"=T3."Enabled" ("禁用")) -> ()  [unwired: 2 in, 2 out]
                n486 = property on="Aquire" class="Bool (strict)"("DisabledEnum"=T3."Disabled and Grayed Out" ("禁用")) -> ()  [unwired: 2 in, 2 out]
                n487 = local write "Aquire"(FALSE ("Initialize")) -> ()
                n488 = property on="Camera Config" class="Bool (strict)"("DisabledEnum"=T3."Disabled and Grayed Out" ("禁用")) -> ()  [unwired: 2 in, 2 out]
                n489 = local read "Binning Enabled"() -> (w211:bool)
                n490 = local read "Binning"() -> (w210:u8[])
                n491 = case shown="False" w211 {
                  tunnel: w210 -> [_ w233]
                  tunnel: [w230 w232] -> w207
                  tunnel: [w230 w231] -> w208
                  frame False {
                    w230 = u8 1 ("Numeric")
                  }
                  frame True {
                    n492 = Index Array(array=w233) -> (element #1=w231:u8, element #2=w232:u8)  [unwired: 2 in]
                  }
                }
                n493 = Divide(x=w206, y=w207) -> (x/y=w204:dbl[])
                n494 = Divide(x=w209, y=w208) -> (x/y=w205:dbl[])
                n495 = Divide(x=w204, y=w205) -> (x/y=w217:dbl[])
                n496 = Array Max & Min(array=w204) -> (max value=w212:dbl)  [unwired: 3 out]
                n497 = Array Max & Min(array=w205) -> (max value=w213:dbl)  [unwired: 3 out]
                n498 = Array Max & Min(array=w217) -> (max index (indices)=w216:i32)  [unwired: 3 out]
                n499 = Greater?(x=w216, y=w214) -> (0:w215:bool)
                n500 = case shown="True" w215 {
                  tunnel: w212 -> [_ _]
                  tunnel: w214 -> [w236 w239]
                  tunnel: w213 -> [w234 w237]
                  frame False {
                    n501 = Multiply(x=w234, y=w236) -> (x*y=w235:dbl)
                    n502 = property on="OD image" class="IntGraph (strict)"("XScale.Maximum"=w235) -> ()  [unwired: 2 in, 2 out]
                    n503 = property on="OD image" class="IntGraph (strict)"("YScale.Maximum"=w234) -> ()  [unwired: 2 in, 2 out]
                  }
                  frame True {
                    n504 = Divide(x=w237, y=w239) -> (x/y=w238:dbl)
                    n505 = property on="OD image" class="IntGraph (strict)"("YScale.Maximum"=w238) -> ()  [unwired: 2 in, 2 out]
                    n506 = property on="OD image" class="IntGraph (strict)"("XScale.Maximum"=w237) -> ()  [unwired: 2 in, 2 out]
                  }
                }
              }
              frame "STOP" {
                w292 = T3."Enabled" ("禁用")
                # "stop the camera"
                n507 = local write "Stop"(FALSE ("Initialize")) -> ()
                n508 = property on="Aquire" class="Bool (strict)"("DisabledEnum"=w292) -> ()  [unwired: 2 in, 2 out]
                n509 = property on="Camera Config" class="Bool (strict)"("DisabledEnum"=w292) -> ()  [unwired: 2 in, 2 out]
                n510 = case shown="False" w284 {
                  tunnel: [w293 w296] -> w286
                  tunnel: w285 -> [w293 w294]
                  frame False {
                  }
                  frame True {
                    n511 = property class="IActiveFlyCapControl"(reference=w294, "Start"=0) -> (reference out=w296:refnum<k7>)  [unwired: 1 in, 1 out]
                  }
                }
                n512 = property class="IActiveFlyCapControl"(reference=w288, "Start"=0) -> (reference out=w287:refnum<k7>)  [unwired: 1 in, 1 out]
                n513 = property on="Stop" class="Bool (strict)"("DisabledEnum"=T3."Disabled and Grayed Out" ("禁用")) -> ()  [unwired: 2 in, 2 out]
              }
              frame "FIT" {
                n514 = stacked-sequence {
                  seq-local: [w300 _ _] -> [_ _ w351]
                  seq-local: [w301 _ _] -> [_ w326 w354]
                  seq-local: [w299 _ _] -> [_ w325 w352]
                  frame #0 {
                    n515 = flat-sequence {
                      tunnel: [w316] -> w301
                      tunnel: [w311] -> w300
                      tunnel: [w310] -> w299
                      frame #0 {
                        # "Fit the latest data"
                        n516 = local read "Latest image data"() -> (w316:dbl[][])
                        n517 = local read "Initial guess values"() -> (w313:dbl[])
                        n518 = local read "Force Guess?"() -> (w314:bool)
                        n519 = local read "Fitting Type"() -> (w315:u16)
                        n520 = vi-ref "fitting modified.vi"() -> (w309:refnum<vi>)
                        n521 = property class="VI"(reference=w309) -> ("Name"=w318:string)  [unwired: 1 in, 2 out]
                        n522 = Open VI Reference(type specifier VI Refnum (for type only)=refnum<vi> refnum, vi path=w318, options=256) -> (vi reference=w308:refnum<vi>)  [unwired: 3 in, 1 out]
                        n523 = call-by-ref "Start Asynchronous Call"(reference=w308, "fitting type"=w315, "2D data"=w316, "force guess?"=w314, "intial guess value"=w313) -> (reference out=w307:refnum<vi>)  [unwired: 9 in, 5 out]
                        n524 = call-by-ref "Wait On Asynchronous Call"(reference=w307) -> (reference out=w312:refnum<vi>, error out=w304:errorcluster, "number of function calls"=w302:i32, "best fit"=w311:dbl[][], "best fit parameters"=w310:dbl[])  [unwired: 13 in, 1 out]
                        n525 = call <vilib>:"Clear Errors.vi"("error in (no error)"=w304, "specific error code to clear (0: all)"=0) -> ()  [unwired: 4 in, 2 out]
                        n526 = Close Reference(reference=w312) -> ()  [unwired: 1 in, 1 out]
                        n527 = local write "number of function calls"(w302) -> ()
                        n528 = local write "Fitting..."(TRUE ("Fitting...")) -> ()
                      }
                      frame #1 {
                        n529 = local write "Fit"(FALSE ("Fit")) -> ()
                      }
                    }
                  }
                  frame #1 {
                    # "Save best fit parameters"
                    n530 = local read "Save Fit"() -> (w328:bool)
                    n531 = local read "Fitting Results Save Path"() -> (w336:string[])
                    n532 = local read "Fitting Type"() -> (w323:u16)
                    n533 = local read "From OD fit?"() -> (w335:bool)
                    n534 = case shown="False" w335 {
                      tunnel: [w348 w350] -> w324
                      frame False {
                        n535 = local read "Current File Num"() -> (w349:u16)
                        n536 = Decrement(x=w349) -> (x-1=w348:u16)
                      }
                      frame True {
                        n537 = local read "OD Num 2"() -> (w350:i32)
                      }
                    }
                    n538 = Array Size(array=w325) -> (size(s)=w333:i32)
                    n539 = Quotient & Remainder(x=w333, y=6) -> (floor(x/y)=w330:i32)  [unwired: 1 out]
                    n540 = Reshape Array(w325, w330, 6 ("dimension size")) -> (w334:dbl[][])
                    n541 = case shown="True" w328 {
                      tunnel: w323 -> [_ w347]
                      tunnel: w336 -> [_ w346]
                      tunnel: w324 -> [_ w345]
                      tunnel: w325 -> [_ w344]
                      frame False {
                      }
                      frame True {
                        n542 = call "Save Best Fit Parameters.vi"("Current File Num"=w345, "Best Fit Parameters"=w344, "Fitting Results Save Path"=w346, "Fitting Type"=w347) -> ()  [unwired: 8 in]
                      }
                    }
                    n543 = Transpose 2D Array(2D array=w334) -> (transposed array=→"best fit parameters":dbl[][])
                    n544 = local read "Direct Summing Cluster"() -> (w327:T1)
                    n545 = Unbundle By Name(w327) -> ("Enable Summing"=w321:bool[], "Direct Summing Path Na"=w322:string)
                    n546 = Index Array(array=w321) -> (element=w320:bool)  [unwired: 1 in]
                    n547 = case shown="True" w320 {
                      tunnel: w323 -> [_ w343]
                      tunnel: w324 -> [_ w342]
                      tunnel: w325 -> [_ w341]
                      tunnel: w326 -> [_ w340]
                      tunnel: w322 -> [_ w337]
                      frame False {
                      }
                      frame True {
                        n548 = local read "Na/Rb (0/1)"() -> (w338:u8)
                        n549 = call "DIRECT SUMMING.vi"("Image Data"=w340, "Fitting Results Save Path"=w337, "Best Fit Parameters"=w341, "File Num"=w342, "Fitting Type"=w343, "Two Cameras?"=FALSE, "Na / Rb"=w338) -> ()  [unwired: 8 in, 1 out]
                      }
                    }
                  }
                  frame #2 {
                    # "Draw Comparison"
                    n550 = call "Draw Comparison.vi"("Best Fit Parameters"=w352, "Best Fit"=w351, "Raw Data"=w354) -> ("Horizontal Comparison"=w356:cluster{i32[], dbl[]}[], "Vertical Comparison"=w357:cluster{i32[], dbl[]}[])  [unwired: 6 in]
                    n551 = local write "Fit"(FALSE ("Initialize")) -> ()
                    n552 = local write "Horizontal Fitting"(w356) -> ()
                    n553 = local write "Vertical Fitting"(w357) -> ()
                    n554 = local write "Fitting..."(FALSE ("Fit Done")) -> ()
                  }
                }
              }
              frame "ODF" {
                w366 = 1.3411 ("y")
                w391 = T5 7 items=["Grayscale (U8)", "Grayscale (I16)", "Grayscale (SGL)", "Complex (CSG)", "RGB (U32)", "HSL (U32)", "RGB (U64)", "Grayscale (U16)"] ("Image Type")
                w384 = "\\" ("字符串")
                n555 = call "find time.vi"() -> ("day"=w382:string, "month"=w379:string, "year"=w376:string)  [unwired: 3 in]
                n556 = Concatenate Strings("D:\\data\\", w376) -> (w377:string)
                n557 = case shown="1" "Open Na/Rb" {
                  tunnel: ["-Na" ("字符串") "-Rb" ("字符串")] -> w358
                  frame 0, Default {
                  }
                  frame 1 {
                  }
                }
                n558 = Less?(x="OD Num", y=100.0) -> (x < y?=w388:bool)
                n559 = Concatenate Strings(w377, w384) -> (w378:string)
                n560 = case shown="True" w388 {
                  tunnel: "OD Num" -> [w410 w412]
                  tunnel: [w409 w411] -> w389
                  frame False {
                    n561 = Number To Decimal String(number=w410) -> (decimal integer string=w409:string)  [unwired: 1 in]
                  }
                  frame True {
                    n562 = Less?(x=w412, y=10.0) -> (x < y?=w413:bool)
                    n563 = case shown="False" w413 {
                      tunnel: w412 -> [w417 w422]
                      tunnel: [w415 w419] -> w411
                      frame False {
                        n564 = Number To Decimal String(number=w417) -> (decimal integer string=w416:string)  [unwired: 1 in]
                        n565 = Concatenate Strings("0" ("字符串"), w416) -> (w415:string)
                      }
                      frame True {
                        n566 = Number To Decimal String(number=w422) -> (decimal integer string=w420:string)  [unwired: 1 in]
                        n567 = Concatenate Strings("00" ("字符串"), w420) -> (w419:string)
                      }
                    }
                  }
                }
                n568 = Concatenate Strings(w378, w379) -> (w380:string)
                n569 = Concatenate Strings(w380, w384) -> (w381:string)
                n570 = Concatenate Strings(w381, w382) -> (w383:string)
                n571 = Concatenate Strings(w383, w384) -> (w385:string)
                n572 = case shown="2" "Ring" {
                  tunnel: ["-1.tif" ("字符串") "-2.tif" ("字符串") "-3.tif" ("字符串") "-OD.tif" ("字符串")] -> w360
                  frame 0, Default {
                  }
                  frame 1 {
                  }
                  frame 2 {
                  }
                  frame 3 {
                  }
                }
                n573 = Concatenate Strings(w385, w389) -> (w386:string)
                n574 = Concatenate Strings(w386, w358) -> (w359:string)
                n575 = Concatenate Strings(w359, w360) -> (w361:string)
                n576 = String To Path(string=w361) -> (path=w394:path)
                n577 = local write "From OD fit?"(TRUE ("From OD fit?")) -> ()
                n578 = local write "OD fit"(FALSE ("OD fit")) -> ()
                n579 = call "IMAQ Create"("Image Name"="untitled", "Image Type"=w391) -> ("New Image"=w395:T6)  [unwired: 3 in, 1 out]
                n580 = call <vilib>:"Open a Document on Disk.vi"("document path"=w394) -> ()  [unwired: 6 in, 1 out]
                n581 = call "IMAQ ReadFile"("File Path"=w394, "Image"=w395) -> ("Image Out"=w396:T6)  [unwired: 5 in, 4 out]
                n582 = call "IMAQ ImageToArray"("Image"=w396) -> ("Image Pixels (U16)"=w370:u16[][], "error out"=w392:errorcluster)  [unwired: 3 in, 3 out]
                n583 = local write "Latest image data"(w370) -> ()
                n584 = Array Size(array=w370) -> (size(s)=w369:i32[])
                n585 = local write "OD image"(w370) -> ()
                n586 = Index Array(array=w369) -> (element #1=w365:i32, element #2=w364:i32)  [unwired: 2 in]
                n587 = Divide(x=w364, y=w365) -> (x/y=w368:dbl)
                n588 = call "IMAQ Dispose"("Image"=w396, "error in (no error)"=w392) -> ()  [unwired: 4 in, 1 out]
                n589 = Greater?(x=w368, y=w366) -> (0:w367:bool)
                n590 = case shown="False" w367 {
                  tunnel: w364 -> [_ w408]
                  tunnel: w366 -> [w405 w407]
                  tunnel: w365 -> [w403 _]
                  frame False {
                    n591 = Multiply(x=w403, y=w405) -> (x*y=w404:dbl)
                    n592 = property on="OD image" class="IntGraph (strict)"("XScale.Maximum"=w404) -> ()  [unwired: 2 in, 2 out]
                    n593 = property on="OD image" class="IntGraph (strict)"("YScale.Maximum"=w403) -> ()  [unwired: 2 in, 2 out]
                  }
                  frame True {
                    n594 = Divide(x=w408, y=w407) -> (x/y=w406:dbl)
                    n595 = property on="OD image" class="IntGraph (strict)"("XScale.Maximum"=w408) -> ()  [unwired: 2 in, 2 out]
                    n596 = property on="OD image" class="IntGraph (strict)"("YScale.Maximum"=w406) -> ()  [unwired: 2 in, 2 out]
                  }
                }
                "OD Num 2" <- "OD Num"
              }
              frame "INI" {
                n597 = Boolean To (0,1)(Boolean=w426) -> (0, 1=w428:i16)
                n598 = Increment(x=w428) -> (x+1=w427:i16)
                n599 = property on="Camera Config" class="Bool (strict)"("DisabledEnum"=T3."Enabled" ("禁用")) -> ()  [unwired: 2 in, 2 out]
                n600 = for {
                  N: w427 -> [_]
                  tunnel: w429 -> [w437]
                  tunnel: w425 -> [w435]
                  tunnel: [w434] -> w424
                  tunnel: [w433] -> w423
                  i -> [w436]
                  n601 = case shown="0, Default" w436 {
                    selector: w436 -> [w441 w449]
                    tunnel: [w438 w450] -> w434
                    tunnel: w437 -> [w440 w447]
                    tunnel: w435 -> [w438 w448]
                    tunnel: [w439 w447] -> w433
                    frame 0, Default {
                      w442 = 1 items=["FreeRunning", "LockNext", "LockLatest"] ("mode")
                      # "Setup Camera Index"
                      # "Set grab mode"
                      # "Make Sure the camera is not running"
                      n602 = property class="IActiveFlyCapControl"(reference=w440, "Camera"=w441) -> (reference out=w443:refnum<k7>)  [unwired: 1 in, 1 out]
                      n603 = invoke class="IActiveFlyCapControl" method="ShowCamSlnModal"(reference=w443) -> (reference out=w445:refnum<k7>)  [unwired: 2 in, 2 out]
                      n604 = property class="IActiveFlyCapControl"(reference=w445, "Start"=0 ("Camera")) -> (reference out=w446:refnum<k7>)  [unwired: 1 in, 1 out]
                      n605 = invoke class="IActiveFlyCapControl" method="SetGrabMode"(reference=w446, "mode"=w442) -> (reference out=w439:refnum<k7>)  [unwired: 2 in, 3 out]
                    }
                    frame 1 {
                      w451 = 1 items=["FreeRunning", "LockNext", "LockLatest"] ("mode")
                      # "Setup Camera Index"
                      # "Set grab mode"
                      # "Make Sure the camera is not running"
                      n606 = property class="IActiveFlyCapControl"(reference=w448, "Camera"=w449) -> (reference out=w452:refnum<k7>)  [unwired: 1 in, 1 out]
                      n607 = invoke class="IActiveFlyCapControl" method="ShowCamSlnModal"(reference=w452) -> (reference out=w454:refnum<k7>)  [unwired: 2 in, 2 out]
                      n608 = property class="IActiveFlyCapControl"(reference=w454, "Start"=0 ("Camera")) -> (reference out=w455:refnum<k7>)  [unwired: 1 in, 1 out]
                      n609 = invoke class="IActiveFlyCapControl" method="SetGrabMode"(reference=w455, "mode"=w451) -> (reference out=w450:refnum<k7>)  [unwired: 2 in, 3 out]
                    }
                  }
                }
                n610 = local write "Initialize"(FALSE ("Initialize")) -> ()
                n611 = property on="Aquire" class="Bool (strict)"("DisabledEnum"=T3."Enabled" ("禁用")) -> ()  [unwired: 2 in, 2 out]
              }
              frame "CLE" {
                n612 = case shown="True" w458 {
                  tunnel: w461 -> [w466 w474]
                  tunnel: [w462 w472] -> w460
                  tunnel: w457 -> [w464 w471]
                  tunnel: [w465 w470] -> w456
                  frame False {
                    n613 = for {
                      N: 5 -> [_]
                      tunnel: [w469] -> w462
                      tunnel: w466 -> [w468]
                      tunnel: [w467] -> w465
                      tunnel: w464 -> [w467]
                      n614 = invoke class="IActiveFlyCapControl" method="GrabImage"(reference=w468) -> (reference out=w469:refnum<k7>)  [unwired: 2 in, 2 out]
                    }
                  }
                  frame True {
                    n615 = for {
                      N: 5 -> [_]
                      tunnel: w474 -> [w478]
                      tunnel: [w477] -> w472
                      tunnel: w471 -> [w476]
                      tunnel: [w475] -> w470
                      n616 = invoke class="IActiveFlyCapControl" method="GrabImage"(reference=w478) -> (reference out=w477:refnum<k7>)  [unwired: 2 in, 2 out]
                      n617 = invoke class="IActiveFlyCapControl" method="GrabImage"(reference=w476) -> (reference out=w475:refnum<k7>)  [unwired: 2 in, 2 out]
                    }
                  }
                }
                n618 = local write "Reset Cam Buffer"(FALSE ("Reset process index")) -> ()
              }
            }
          }
        }
        n619 = Wait Until Next ms Multiple(millisecond multiple=u32 100) -> ()  [unwired: 1 out]
        n620 = local read "Exit"() -> (w110:bool)
      }
    }
    frame #2 {
      n621 = Release Queue(queue=w1225) -> ()  [unwired: 2 in, 3 out]
      n622 = Release Queue(queue=w1227) -> ()  [unwired: 2 in, 3 out]
      n623 = Release Queue(queue=w1226) -> ()  [unwired: 2 in, 3 out]
    }
  }
